vi "tiffWriteTags.vi"(6 "BitsPerSample":i32, 7 "Compress?":bool=TRUE, 8 "ImageDescription":string, 9 "Multipage":cluster{"Page":i32, "TotalPages":i32}, 10 "Dimensions":T1, 11 "TiffIn":refnum<k24>) -> (3 "TiffOut":refnum<k24>)   [LabVIEW 2012, in "LVTiffWriter.lvlib"]
uses:
  LVTiffWriter.lvlib
  D:/MyDocuments/LabVIEW Data/SPIM/Shared/libtiff.net_bin-2.4.500.0/BitMiracle.LibTiff.NET.dll
  BitMiracle.LibTiff.NET.dll
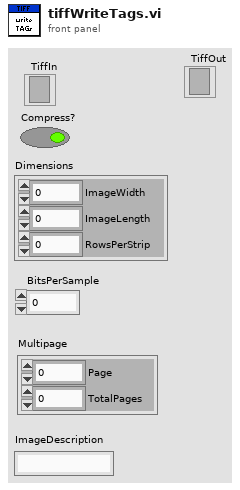
[diagram p1: front panel]
types:
  T1 = cluster{"ImageWidth":i32, "ImageLength":i32, "RowsPerStrip":i32}
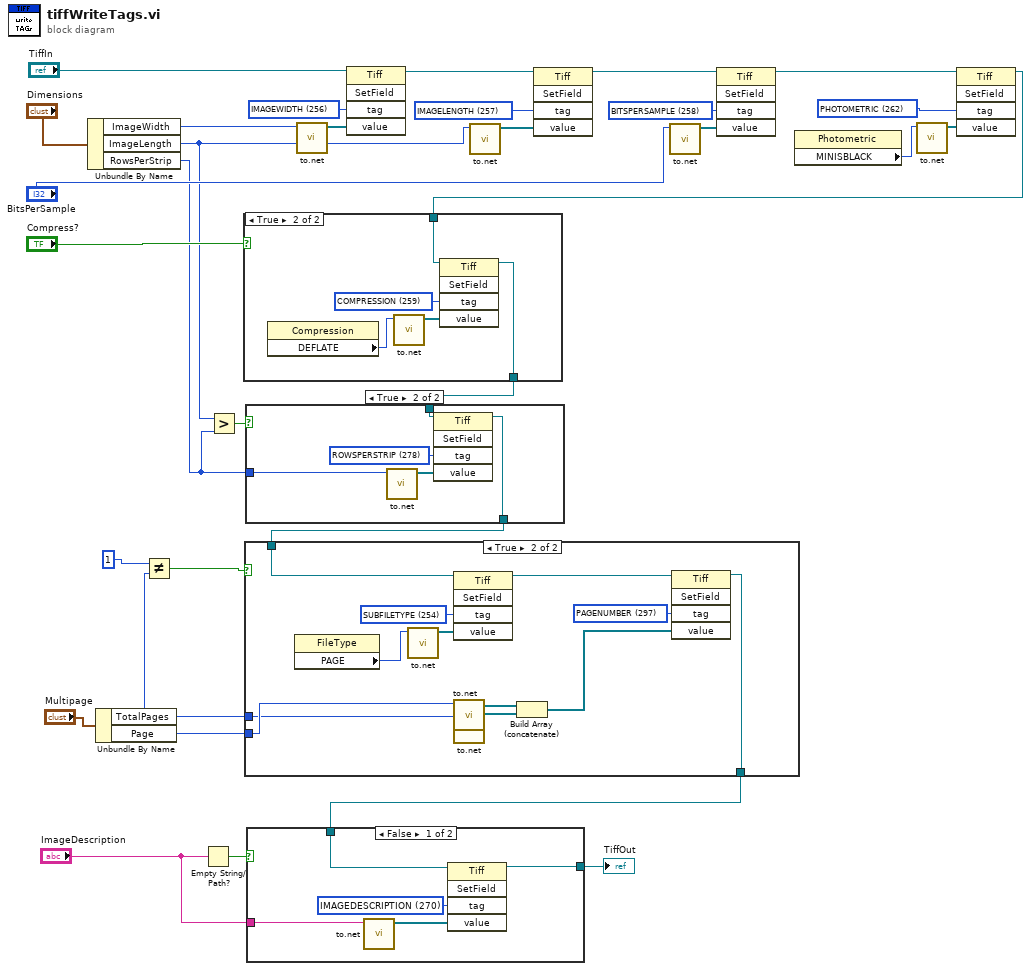
[diagram p0: block diagram]
diagram:
  w28 = 262 items=["IGNORE"=0, "SUBFILETYPE"=254, "OSUBFILETYPE"=255, "IMAGEWIDTH"=256, "IMAGELENGTH"=257, "BITSPERSAMPLE"=258, "COMPRESSION"=259, "PHOTOMETRIC"=262, "THRESHHOLDING"=263, "CELLWIDTH"=264, "CELLLENGTH"=265, "FILLORDER"=266, "DOCUMENTNAME"=269, "IMAGEDESCRIPTION"=270, "MAKE"=271, "MODEL"=272, "STRIPOFFSETS"=273, "ORIENTATION"=274, "SAMPLESPERPIXEL"=277, "ROWSPERSTRIP"=278, "STRIPBYTECOUNTS"=279, "MINSAMPLEVALUE"=280, "MAXSAMPLEVALUE"=281, "XRESOLUTION"=282, "YRESOLUTION"=283, "PLANARCONFIG"=284, "PAGENAME"=285, "XPOSITION"=286, "YPOSITION"=287, "FREEOFFSETS"=288, "FREEBYTECOUNTS"=289, "GRAYRESPONSEUNIT"=290, "GRAYRESPONSECURVE"=291, "GROUP3OPTIONS, T4OPTIONS"=292, "GROUP4OPTIONS, T6OPTIONS"=293, "RESOLUTIONUNIT"=296, "PAGENUMBER"=297, "COLORRESPONSEUNIT"=300, "TRANSFERFUNCTION"=301, "SOFTWARE"=305, "DATETIME"=306, "ARTIST"=315, "HOSTCOMPUTER"=316, "PREDICTOR"=317, "WHITEPOINT"=318, "PRIMARYCHROMATICITIES"=319, "COLORMAP"=320, "HALFTONEHINTS"=321, "TILEWIDTH"=322, "TILELENGTH"=323, "TILEOFFSETS"=324, "TILEBYTECOUNTS"=325, "BADFAXLINES"=326, "CLEANFAXDATA"=327, "CONSECUTIVEBADFAXLINES"=328, "SUBIFD"=330, "INKSET"=332, "INKNAMES"=333, "NUMBEROFINKS"=334, "DOTRANGE"=336, "TARGETPRINTER"=337, "EXTRASAMPLES"=338, "SAMPLEFORMAT"=339, "SMINSAMPLEVALUE"=340, "SMAXSAMPLEVALUE"=341, "CLIPPATH"=343, "XCLIPPATHUNITS"=344, "YCLIPPATHUNITS"=345, "INDEXED"=346, "JPEGTABLES"=347, "OPIPROXY"=351, "JPEGPROC"=512, "JPEGIFOFFSET"=513, "JPEGIFBYTECOUNT"=514, "JPEGRESTARTINTERVAL"=515, "JPEGLOSSLESSPREDICTORS"=517, "JPEGPOINTTRANSFORM"=518, "JPEGQTABLES"=519, "JPEGDCTABLES"=520, "JPEGACTABLES"=521, "YCBCRCOEFFICIENTS"=529, "YCBCRSUBSAMPLING"=530, "YCBCRPOSITIONING"=531, "REFERENCEBLACKWHITE"=532, "XMLPACKET"=700, "OPIIMAGEID"=32781, "REFPTS"=32953, "REGIONTACKPOINT"=32954, "REGIONWARPCORNERS"=32955, "REGIONAFFINE"=32956, "MATTEING"=32995, "DATATYPE"=32996, "IMAGEDEPTH"=32997, "TILEDEPTH"=32998, "PIXAR_IMAGEFULLWIDTH"=33300, "PIXAR_IMAGEFULLLENGTH"=33301, "PIXAR_TEXTUREFORMAT"=33302, "PIXAR_WRAPMODES"=33303, "PIXAR_FOVCOT"=33304, "PIXAR_MATRIX_WORLDTOSCREEN"=33305, "PIXAR_MATRIX_WORLDTOCAMERA"=33306, "WRITERSERIALNUMBER"=33405, "COPYRIGHT"=33432, "EXIF_EXPOSURETIME"=33434, "EXIF_FNUMBER"=33437, "RICHTIFFIPTC"=33723, "IT8SITE"=34016, "IT8COLORSEQUENCE"=34017, "IT8HEADER"=34018, "IT8RASTERPADDING"=34019, "IT8BITSPERRUNLENGTH"=34020, "IT8BITSPEREXTENDEDRUNLENGTH"=34021, "IT8COLORTABLE"=34022, "IT8IMAGECOLORINDICATOR"=34023, "IT8BKGCOLORINDICATOR"=34024, "IT8IMAGECOLORVALUE"=34025, "IT8BKGCOLORVALUE"=34026, "IT8PIXELINTENSITYRANGE"=34027, "IT8TRANSPARENCYINDICATOR"=34028, "IT8COLORCHARACTERIZATION"=34029, "IT8HCUSAGE"=34030, "IT8TRAPINDICATOR"=34031, "IT8CMYKEQUIVALENT"=34032, "FRAMECOUNT"=34232, "PHOTOSHOP"=34377, "EXIFIFD"=34665, "ICCPROFILE"=34675, "JBIGOPTIONS"=34750, "EXIF_EXPOSUREPROGRAM"=34850, "EXIF_SPECTRALSENSITIVITY"=34852, "GPSIFD"=34853, "EXIF_ISOSPEEDRATINGS"=34855, "EXIF_OECF"=34856, "FAXRECVPARAMS"=34908, "FAXSUBADDRESS"=34909, "FAXRECVTIME"=34910, "FAXDCS"=34911, "FEDEX_EDR"=34929, "EXIF_EXIFVERSION"=36864, "EXIF_DATETIMEORIGINAL"=36867, "EXIF_DATETIMEDIGITIZED"=36868, "EXIF_COMPONENTSCONFIGURATION"=37121, "EXIF_COMPRESSEDBITSPERPIXEL"=37122, "EXIF_SHUTTERSPEEDVALUE"=37377, "EXIF_APERTUREVALUE"=37378, "EXIF_BRIGHTNESSVALUE"=37379, "EXIF_EXPOSUREBIASVALUE"=37380, "EXIF_MAXAPERTUREVALUE"=37381, "EXIF_SUBJECTDISTANCE"=37382, "EXIF_METERINGMODE"=37383, "EXIF_LIGHTSOURCE"=37384, "EXIF_FLASH"=37385, "EXIF_FOCALLENGTH"=37386, "EXIF_SUBJECTAREA"=37396, "STONITS"=37439, "EXIF_MAKERNOTE"=37500, "EXIF_USERCOMMENT"=37510, "EXIF_SUBSECTIME"=37520, "EXIF_SUBSECTIMEORIGINAL"=37521, "EXIF_SUBSECTIMEDIGITIZED"=37522, "EXIF_FLASHPIXVERSION"=40960, "EXIF_COLORSPACE"=40961, "EXIF_PIXELXDIMENSION"=40962, "EXIF_PIXELYDIMENSION"=40963, "EXIF_RELATEDSOUNDFILE"=40964, "INTEROPERABILITYIFD"=40965, "EXIF_FLASHENERGY"=41483, "EXIF_SPATIALFREQUENCYRESPONSE"=41484, "EXIF_FOCALPLANEXRESOLUTION"=41486, "EXIF_FOCALPLANEYRESOLUTION"=41487, "EXIF_FOCALPLANERESOLUTIONUNIT"=41488, "EXIF_SUBJECTLOCATION"=41492, "EXIF_EXPOSUREINDEX"=41493, "EXIF_SENSINGMETHOD"=41495, "EXIF_FILESOURCE"=41728, "EXIF_SCENETYPE"=41729, "EXIF_CFAPATTERN"=41730, "EXIF_CUSTOMRENDERED"=41985, "EXIF_EXPOSUREMODE"=41986, "EXIF_WHITEBALANCE"=41987, "EXIF_DIGITALZOOMRATIO"=41988, "EXIF_FOCALLENGTHIN35MMFILM"=41989, "EXIF_SCENECAPTURETYPE"=41990, "EXIF_GAINCONTROL"=41991, "EXIF_CONTRAST"=41992, "EXIF_SATURATION"=41993, "EXIF_SHARPNESS"=41994, "EXIF_DEVICESETTINGDESCRIPTION"=41995, "EXIF_SUBJECTDISTANCERANGE"=41996, "EXIF_IMAGEUNIQUEID"=42016, "DNGVERSION"=50706, "DNGBACKWARDVERSION"=50707, "UNIQUECAMERAMODEL"=50708, "LOCALIZEDCAMERAMODEL"=50709, "CFAPLANECOLOR"=50710, "CFALAYOUT"=50711, "LINEARIZATIONTABLE"=50712, "BLACKLEVELREPEATDIM"=50713, "BLACKLEVEL"=50714, "BLACKLEVELDELTAH"=50715, "BLACKLEVELDELTAV"=50716, "WHITELEVEL"=50717, "DEFAULTSCALE"=50718, "DEFAULTCROPORIGIN"=50719, "DEFAULTCROPSIZE"=50720, "COLORMATRIX1"=50721, "COLORMATRIX2"=50722, "CAMERACALIBRATION1"=50723, "CAMERACALIBRATION2"=50724, "REDUCTIONMATRIX1"=50725, "REDUCTIONMATRIX2"=50726, "ANALOGBALANCE"=50727, "ASSHOTNEUTRAL"=50728, "ASSHOTWHITEXY"=50729, "BASELINEEXPOSURE"=50730, "BASELINENOISE"=50731, "BASELINESHARPNESS"=50732, "BAYERGREENSPLIT"=50733, "LINEARRESPONSELIMIT"=50734, "CAMERASERIALNUMBER"=50735, "LENSINFO"=50736, "CHROMABLURRADIUS"=50737, "ANTIALIASSTRENGTH"=50738, "SHADOWSCALE"=50739, "DNGPRIVATEDATA"=50740, "MAKERNOTESAFETY"=50741, "CALIBRATIONILLUMINANT1"=50778, "CALIBRATIONILLUMINANT2"=50779, "BESTQUALITYSCALE"=50780, "RAWDATAUNIQUEID"=50781, "ORIGINALRAWFILENAME"=50827, "ORIGINALRAWFILEDATA"=50828, "ACTIVEAREA"=50829, "MASKEDAREAS"=50830, "ASSHOTICCPROFILE"=50831, "ASSHOTPREPROFILEMATRIX"=50832, "CURRENTICCPROFILE"=50833, "CURRENTPREPROFILEMATRIX"=50834, "DCSHUESHIFTVALUES"=65535, "FAXMODE"=65536, "JPEGQUALITY"=65537, "JPEGCOLORMODE"=65538, "JPEGTABLESMODE"=65539, "FAXFILLFUNC"=65540, "PIXARLOGDATAFMT"=65549, "DCSIMAGERTYPE"=65550, "DCSINTERPMODE"=65551, "DCSBALANCEARRAY"=65552, "DCSCORRECTMATRIX"=65553, "DCSGAMMA"=65554, "DCSTOESHOULDERPTS"=65555, "DCSCALIBRATIONFD"=65556, "ZIPQUALITY"=65557, "PIXARLOGQUALITY"=65558, "DCSCLIPRECTANGLE"=65559, "SGILOGDATAFMT"=65560, "SGILOGENCODE"=65561] ("tag")
  w26 = 258 items=["IGNORE"=0, "SUBFILETYPE"=254, "OSUBFILETYPE"=255, "IMAGEWIDTH"=256, "IMAGELENGTH"=257, "BITSPERSAMPLE"=258, "COMPRESSION"=259, "PHOTOMETRIC"=262, "THRESHHOLDING"=263, "CELLWIDTH"=264, "CELLLENGTH"=265, "FILLORDER"=266, "DOCUMENTNAME"=269, "IMAGEDESCRIPTION"=270, "MAKE"=271, "MODEL"=272, "STRIPOFFSETS"=273, "ORIENTATION"=274, "SAMPLESPERPIXEL"=277, "ROWSPERSTRIP"=278, "STRIPBYTECOUNTS"=279, "MINSAMPLEVALUE"=280, "MAXSAMPLEVALUE"=281, "XRESOLUTION"=282, "YRESOLUTION"=283, "PLANARCONFIG"=284, "PAGENAME"=285, "XPOSITION"=286, "YPOSITION"=287, "FREEOFFSETS"=288, "FREEBYTECOUNTS"=289, "GRAYRESPONSEUNIT"=290, "GRAYRESPONSECURVE"=291, "GROUP3OPTIONS, T4OPTIONS"=292, "GROUP4OPTIONS, T6OPTIONS"=293, "RESOLUTIONUNIT"=296, "PAGENUMBER"=297, "COLORRESPONSEUNIT"=300, "TRANSFERFUNCTION"=301, "SOFTWARE"=305, "DATETIME"=306, "ARTIST"=315, "HOSTCOMPUTER"=316, "PREDICTOR"=317, "WHITEPOINT"=318, "PRIMARYCHROMATICITIES"=319, "COLORMAP"=320, "HALFTONEHINTS"=321, "TILEWIDTH"=322, "TILELENGTH"=323, "TILEOFFSETS"=324, "TILEBYTECOUNTS"=325, "BADFAXLINES"=326, "CLEANFAXDATA"=327, "CONSECUTIVEBADFAXLINES"=328, "SUBIFD"=330, "INKSET"=332, "INKNAMES"=333, "NUMBEROFINKS"=334, "DOTRANGE"=336, "TARGETPRINTER"=337, "EXTRASAMPLES"=338, "SAMPLEFORMAT"=339, "SMINSAMPLEVALUE"=340, "SMAXSAMPLEVALUE"=341, "CLIPPATH"=343, "XCLIPPATHUNITS"=344, "YCLIPPATHUNITS"=345, "INDEXED"=346, "JPEGTABLES"=347, "OPIPROXY"=351, "JPEGPROC"=512, "JPEGIFOFFSET"=513, "JPEGIFBYTECOUNT"=514, "JPEGRESTARTINTERVAL"=515, "JPEGLOSSLESSPREDICTORS"=517, "JPEGPOINTTRANSFORM"=518, "JPEGQTABLES"=519, "JPEGDCTABLES"=520, "JPEGACTABLES"=521, "YCBCRCOEFFICIENTS"=529, "YCBCRSUBSAMPLING"=530, "YCBCRPOSITIONING"=531, "REFERENCEBLACKWHITE"=532, "XMLPACKET"=700, "OPIIMAGEID"=32781, "REFPTS"=32953, "REGIONTACKPOINT"=32954, "REGIONWARPCORNERS"=32955, "REGIONAFFINE"=32956, "MATTEING"=32995, "DATATYPE"=32996, "IMAGEDEPTH"=32997, "TILEDEPTH"=32998, "PIXAR_IMAGEFULLWIDTH"=33300, "PIXAR_IMAGEFULLLENGTH"=33301, "PIXAR_TEXTUREFORMAT"=33302, "PIXAR_WRAPMODES"=33303, "PIXAR_FOVCOT"=33304, "PIXAR_MATRIX_WORLDTOSCREEN"=33305, "PIXAR_MATRIX_WORLDTOCAMERA"=33306, "WRITERSERIALNUMBER"=33405, "COPYRIGHT"=33432, "EXIF_EXPOSURETIME"=33434, "EXIF_FNUMBER"=33437, "RICHTIFFIPTC"=33723, "IT8SITE"=34016, "IT8COLORSEQUENCE"=34017, "IT8HEADER"=34018, "IT8RASTERPADDING"=34019, "IT8BITSPERRUNLENGTH"=34020, "IT8BITSPEREXTENDEDRUNLENGTH"=34021, "IT8COLORTABLE"=34022, "IT8IMAGECOLORINDICATOR"=34023, "IT8BKGCOLORINDICATOR"=34024, "IT8IMAGECOLORVALUE"=34025, "IT8BKGCOLORVALUE"=34026, "IT8PIXELINTENSITYRANGE"=34027, "IT8TRANSPARENCYINDICATOR"=34028, "IT8COLORCHARACTERIZATION"=34029, "IT8HCUSAGE"=34030, "IT8TRAPINDICATOR"=34031, "IT8CMYKEQUIVALENT"=34032, "FRAMECOUNT"=34232, "PHOTOSHOP"=34377, "EXIFIFD"=34665, "ICCPROFILE"=34675, "JBIGOPTIONS"=34750, "EXIF_EXPOSUREPROGRAM"=34850, "EXIF_SPECTRALSENSITIVITY"=34852, "GPSIFD"=34853, "EXIF_ISOSPEEDRATINGS"=34855, "EXIF_OECF"=34856, "FAXRECVPARAMS"=34908, "FAXSUBADDRESS"=34909, "FAXRECVTIME"=34910, "FAXDCS"=34911, "FEDEX_EDR"=34929, "EXIF_EXIFVERSION"=36864, "EXIF_DATETIMEORIGINAL"=36867, "EXIF_DATETIMEDIGITIZED"=36868, "EXIF_COMPONENTSCONFIGURATION"=37121, "EXIF_COMPRESSEDBITSPERPIXEL"=37122, "EXIF_SHUTTERSPEEDVALUE"=37377, "EXIF_APERTUREVALUE"=37378, "EXIF_BRIGHTNESSVALUE"=37379, "EXIF_EXPOSUREBIASVALUE"=37380, "EXIF_MAXAPERTUREVALUE"=37381, "EXIF_SUBJECTDISTANCE"=37382, "EXIF_METERINGMODE"=37383, "EXIF_LIGHTSOURCE"=37384, "EXIF_FLASH"=37385, "EXIF_FOCALLENGTH"=37386, "EXIF_SUBJECTAREA"=37396, "STONITS"=37439, "EXIF_MAKERNOTE"=37500, "EXIF_USERCOMMENT"=37510, "EXIF_SUBSECTIME"=37520, "EXIF_SUBSECTIMEORIGINAL"=37521, "EXIF_SUBSECTIMEDIGITIZED"=37522, "EXIF_FLASHPIXVERSION"=40960, "EXIF_COLORSPACE"=40961, "EXIF_PIXELXDIMENSION"=40962, "EXIF_PIXELYDIMENSION"=40963, "EXIF_RELATEDSOUNDFILE"=40964, "INTEROPERABILITYIFD"=40965, "EXIF_FLASHENERGY"=41483, "EXIF_SPATIALFREQUENCYRESPONSE"=41484, "EXIF_FOCALPLANEXRESOLUTION"=41486, "EXIF_FOCALPLANEYRESOLUTION"=41487, "EXIF_FOCALPLANERESOLUTIONUNIT"=41488, "EXIF_SUBJECTLOCATION"=41492, "EXIF_EXPOSUREINDEX"=41493, "EXIF_SENSINGMETHOD"=41495, "EXIF_FILESOURCE"=41728, "EXIF_SCENETYPE"=41729, "EXIF_CFAPATTERN"=41730, "EXIF_CUSTOMRENDERED"=41985, "EXIF_EXPOSUREMODE"=41986, "EXIF_WHITEBALANCE"=41987, "EXIF_DIGITALZOOMRATIO"=41988, "EXIF_FOCALLENGTHIN35MMFILM"=41989, "EXIF_SCENECAPTURETYPE"=41990, "EXIF_GAINCONTROL"=41991, "EXIF_CONTRAST"=41992, "EXIF_SATURATION"=41993, "EXIF_SHARPNESS"=41994, "EXIF_DEVICESETTINGDESCRIPTION"=41995, "EXIF_SUBJECTDISTANCERANGE"=41996, "EXIF_IMAGEUNIQUEID"=42016, "DNGVERSION"=50706, "DNGBACKWARDVERSION"=50707, "UNIQUECAMERAMODEL"=50708, "LOCALIZEDCAMERAMODEL"=50709, "CFAPLANECOLOR"=50710, "CFALAYOUT"=50711, "LINEARIZATIONTABLE"=50712, "BLACKLEVELREPEATDIM"=50713, "BLACKLEVEL"=50714, "BLACKLEVELDELTAH"=50715, "BLACKLEVELDELTAV"=50716, "WHITELEVEL"=50717, "DEFAULTSCALE"=50718, "DEFAULTCROPORIGIN"=50719, "DEFAULTCROPSIZE"=50720, "COLORMATRIX1"=50721, "COLORMATRIX2"=50722, "CAMERACALIBRATION1"=50723, "CAMERACALIBRATION2"=50724, "REDUCTIONMATRIX1"=50725, "REDUCTIONMATRIX2"=50726, "ANALOGBALANCE"=50727, "ASSHOTNEUTRAL"=50728, "ASSHOTWHITEXY"=50729, "BASELINEEXPOSURE"=50730, "BASELINENOISE"=50731, "BASELINESHARPNESS"=50732, "BAYERGREENSPLIT"=50733, "LINEARRESPONSELIMIT"=50734, "CAMERASERIALNUMBER"=50735, "LENSINFO"=50736, "CHROMABLURRADIUS"=50737, "ANTIALIASSTRENGTH"=50738, "SHADOWSCALE"=50739, "DNGPRIVATEDATA"=50740, "MAKERNOTESAFETY"=50741, "CALIBRATIONILLUMINANT1"=50778, "CALIBRATIONILLUMINANT2"=50779, "BESTQUALITYSCALE"=50780, "RAWDATAUNIQUEID"=50781, "ORIGINALRAWFILENAME"=50827, "ORIGINALRAWFILEDATA"=50828, "ACTIVEAREA"=50829, "MASKEDAREAS"=50830, "ASSHOTICCPROFILE"=50831, "ASSHOTPREPROFILEMATRIX"=50832, "CURRENTICCPROFILE"=50833, "CURRENTPREPROFILEMATRIX"=50834, "DCSHUESHIFTVALUES"=65535, "FAXMODE"=65536, "JPEGQUALITY"=65537, "JPEGCOLORMODE"=65538, "JPEGTABLESMODE"=65539, "FAXFILLFUNC"=65540, "PIXARLOGDATAFMT"=65549, "DCSIMAGERTYPE"=65550, "DCSINTERPMODE"=65551, "DCSBALANCEARRAY"=65552, "DCSCORRECTMATRIX"=65553, "DCSGAMMA"=65554, "DCSTOESHOULDERPTS"=65555, "DCSCALIBRATIONFD"=65556, "ZIPQUALITY"=65557, "PIXARLOGQUALITY"=65558, "DCSCLIPRECTANGLE"=65559, "SGILOGDATAFMT"=65560, "SGILOGENCODE"=65561] ("tag")
  w23 = 257 items=["IGNORE"=0, "SUBFILETYPE"=254, "OSUBFILETYPE"=255, "IMAGEWIDTH"=256, "IMAGELENGTH"=257, "BITSPERSAMPLE"=258, "COMPRESSION"=259, "PHOTOMETRIC"=262, "THRESHHOLDING"=263, "CELLWIDTH"=264, "CELLLENGTH"=265, "FILLORDER"=266, "DOCUMENTNAME"=269, "IMAGEDESCRIPTION"=270, "MAKE"=271, "MODEL"=272, "STRIPOFFSETS"=273, "ORIENTATION"=274, "SAMPLESPERPIXEL"=277, "ROWSPERSTRIP"=278, "STRIPBYTECOUNTS"=279, "MINSAMPLEVALUE"=280, "MAXSAMPLEVALUE"=281, "XRESOLUTION"=282, "YRESOLUTION"=283, "PLANARCONFIG"=284, "PAGENAME"=285, "XPOSITION"=286, "YPOSITION"=287, "FREEOFFSETS"=288, "FREEBYTECOUNTS"=289, "GRAYRESPONSEUNIT"=290, "GRAYRESPONSECURVE"=291, "GROUP3OPTIONS, T4OPTIONS"=292, "GROUP4OPTIONS, T6OPTIONS"=293, "RESOLUTIONUNIT"=296, "PAGENUMBER"=297, "COLORRESPONSEUNIT"=300, "TRANSFERFUNCTION"=301, "SOFTWARE"=305, "DATETIME"=306, "ARTIST"=315, "HOSTCOMPUTER"=316, "PREDICTOR"=317, "WHITEPOINT"=318, "PRIMARYCHROMATICITIES"=319, "COLORMAP"=320, "HALFTONEHINTS"=321, "TILEWIDTH"=322, "TILELENGTH"=323, "TILEOFFSETS"=324, "TILEBYTECOUNTS"=325, "BADFAXLINES"=326, "CLEANFAXDATA"=327, "CONSECUTIVEBADFAXLINES"=328, "SUBIFD"=330, "INKSET"=332, "INKNAMES"=333, "NUMBEROFINKS"=334, "DOTRANGE"=336, "TARGETPRINTER"=337, "EXTRASAMPLES"=338, "SAMPLEFORMAT"=339, "SMINSAMPLEVALUE"=340, "SMAXSAMPLEVALUE"=341, "CLIPPATH"=343, "XCLIPPATHUNITS"=344, "YCLIPPATHUNITS"=345, "INDEXED"=346, "JPEGTABLES"=347, "OPIPROXY"=351, "JPEGPROC"=512, "JPEGIFOFFSET"=513, "JPEGIFBYTECOUNT"=514, "JPEGRESTARTINTERVAL"=515, "JPEGLOSSLESSPREDICTORS"=517, "JPEGPOINTTRANSFORM"=518, "JPEGQTABLES"=519, "JPEGDCTABLES"=520, "JPEGACTABLES"=521, "YCBCRCOEFFICIENTS"=529, "YCBCRSUBSAMPLING"=530, "YCBCRPOSITIONING"=531, "REFERENCEBLACKWHITE"=532, "XMLPACKET"=700, "OPIIMAGEID"=32781, "REFPTS"=32953, "REGIONTACKPOINT"=32954, "REGIONWARPCORNERS"=32955, "REGIONAFFINE"=32956, "MATTEING"=32995, "DATATYPE"=32996, "IMAGEDEPTH"=32997, "TILEDEPTH"=32998, "PIXAR_IMAGEFULLWIDTH"=33300, "PIXAR_IMAGEFULLLENGTH"=33301, "PIXAR_TEXTUREFORMAT"=33302, "PIXAR_WRAPMODES"=33303, "PIXAR_FOVCOT"=33304, "PIXAR_MATRIX_WORLDTOSCREEN"=33305, "PIXAR_MATRIX_WORLDTOCAMERA"=33306, "WRITERSERIALNUMBER"=33405, "COPYRIGHT"=33432, "EXIF_EXPOSURETIME"=33434, "EXIF_FNUMBER"=33437, "RICHTIFFIPTC"=33723, "IT8SITE"=34016, "IT8COLORSEQUENCE"=34017, "IT8HEADER"=34018, "IT8RASTERPADDING"=34019, "IT8BITSPERRUNLENGTH"=34020, "IT8BITSPEREXTENDEDRUNLENGTH"=34021, "IT8COLORTABLE"=34022, "IT8IMAGECOLORINDICATOR"=34023, "IT8BKGCOLORINDICATOR"=34024, "IT8IMAGECOLORVALUE"=34025, "IT8BKGCOLORVALUE"=34026, "IT8PIXELINTENSITYRANGE"=34027, "IT8TRANSPARENCYINDICATOR"=34028, "IT8COLORCHARACTERIZATION"=34029, "IT8HCUSAGE"=34030, "IT8TRAPINDICATOR"=34031, "IT8CMYKEQUIVALENT"=34032, "FRAMECOUNT"=34232, "PHOTOSHOP"=34377, "EXIFIFD"=34665, "ICCPROFILE"=34675, "JBIGOPTIONS"=34750, "EXIF_EXPOSUREPROGRAM"=34850, "EXIF_SPECTRALSENSITIVITY"=34852, "GPSIFD"=34853, "EXIF_ISOSPEEDRATINGS"=34855, "EXIF_OECF"=34856, "FAXRECVPARAMS"=34908, "FAXSUBADDRESS"=34909, "FAXRECVTIME"=34910, "FAXDCS"=34911, "FEDEX_EDR"=34929, "EXIF_EXIFVERSION"=36864, "EXIF_DATETIMEORIGINAL"=36867, "EXIF_DATETIMEDIGITIZED"=36868, "EXIF_COMPONENTSCONFIGURATION"=37121, "EXIF_COMPRESSEDBITSPERPIXEL"=37122, "EXIF_SHUTTERSPEEDVALUE"=37377, "EXIF_APERTUREVALUE"=37378, "EXIF_BRIGHTNESSVALUE"=37379, "EXIF_EXPOSUREBIASVALUE"=37380, "EXIF_MAXAPERTUREVALUE"=37381, "EXIF_SUBJECTDISTANCE"=37382, "EXIF_METERINGMODE"=37383, "EXIF_LIGHTSOURCE"=37384, "EXIF_FLASH"=37385, "EXIF_FOCALLENGTH"=37386, "EXIF_SUBJECTAREA"=37396, "STONITS"=37439, "EXIF_MAKERNOTE"=37500, "EXIF_USERCOMMENT"=37510, "EXIF_SUBSECTIME"=37520, "EXIF_SUBSECTIMEORIGINAL"=37521, "EXIF_SUBSECTIMEDIGITIZED"=37522, "EXIF_FLASHPIXVERSION"=40960, "EXIF_COLORSPACE"=40961, "EXIF_PIXELXDIMENSION"=40962, "EXIF_PIXELYDIMENSION"=40963, "EXIF_RELATEDSOUNDFILE"=40964, "INTEROPERABILITYIFD"=40965, "EXIF_FLASHENERGY"=41483, "EXIF_SPATIALFREQUENCYRESPONSE"=41484, "EXIF_FOCALPLANEXRESOLUTION"=41486, "EXIF_FOCALPLANEYRESOLUTION"=41487, "EXIF_FOCALPLANERESOLUTIONUNIT"=41488, "EXIF_SUBJECTLOCATION"=41492, "EXIF_EXPOSUREINDEX"=41493, "EXIF_SENSINGMETHOD"=41495, "EXIF_FILESOURCE"=41728, "EXIF_SCENETYPE"=41729, "EXIF_CFAPATTERN"=41730, "EXIF_CUSTOMRENDERED"=41985, "EXIF_EXPOSUREMODE"=41986, "EXIF_WHITEBALANCE"=41987, "EXIF_DIGITALZOOMRATIO"=41988, "EXIF_FOCALLENGTHIN35MMFILM"=41989, "EXIF_SCENECAPTURETYPE"=41990, "EXIF_GAINCONTROL"=41991, "EXIF_CONTRAST"=41992, "EXIF_SATURATION"=41993, "EXIF_SHARPNESS"=41994, "EXIF_DEVICESETTINGDESCRIPTION"=41995, "EXIF_SUBJECTDISTANCERANGE"=41996, "EXIF_IMAGEUNIQUEID"=42016, "DNGVERSION"=50706, "DNGBACKWARDVERSION"=50707, "UNIQUECAMERAMODEL"=50708, "LOCALIZEDCAMERAMODEL"=50709, "CFAPLANECOLOR"=50710, "CFALAYOUT"=50711, "LINEARIZATIONTABLE"=50712, "BLACKLEVELREPEATDIM"=50713, "BLACKLEVEL"=50714, "BLACKLEVELDELTAH"=50715, "BLACKLEVELDELTAV"=50716, "WHITELEVEL"=50717, "DEFAULTSCALE"=50718, "DEFAULTCROPORIGIN"=50719, "DEFAULTCROPSIZE"=50720, "COLORMATRIX1"=50721, "COLORMATRIX2"=50722, "CAMERACALIBRATION1"=50723, "CAMERACALIBRATION2"=50724, "REDUCTIONMATRIX1"=50725, "REDUCTIONMATRIX2"=50726, "ANALOGBALANCE"=50727, "ASSHOTNEUTRAL"=50728, "ASSHOTWHITEXY"=50729, "BASELINEEXPOSURE"=50730, "BASELINENOISE"=50731, "BASELINESHARPNESS"=50732, "BAYERGREENSPLIT"=50733, "LINEARRESPONSELIMIT"=50734, "CAMERASERIALNUMBER"=50735, "LENSINFO"=50736, "CHROMABLURRADIUS"=50737, "ANTIALIASSTRENGTH"=50738, "SHADOWSCALE"=50739, "DNGPRIVATEDATA"=50740, "MAKERNOTESAFETY"=50741, "CALIBRATIONILLUMINANT1"=50778, "CALIBRATIONILLUMINANT2"=50779, "BESTQUALITYSCALE"=50780, "RAWDATAUNIQUEID"=50781, "ORIGINALRAWFILENAME"=50827, "ORIGINALRAWFILEDATA"=50828, "ACTIVEAREA"=50829, "MASKEDAREAS"=50830, "ASSHOTICCPROFILE"=50831, "ASSHOTPREPROFILEMATRIX"=50832, "CURRENTICCPROFILE"=50833, "CURRENTPREPROFILEMATRIX"=50834, "DCSHUESHIFTVALUES"=65535, "FAXMODE"=65536, "JPEGQUALITY"=65537, "JPEGCOLORMODE"=65538, "JPEGTABLESMODE"=65539, "FAXFILLFUNC"=65540, "PIXARLOGDATAFMT"=65549, "DCSIMAGERTYPE"=65550, "DCSINTERPMODE"=65551, "DCSBALANCEARRAY"=65552, "DCSCORRECTMATRIX"=65553, "DCSGAMMA"=65554, "DCSTOESHOULDERPTS"=65555, "DCSCALIBRATIONFD"=65556, "ZIPQUALITY"=65557, "PIXARLOGQUALITY"=65558, "DCSCLIPRECTANGLE"=65559, "SGILOGDATAFMT"=65560, "SGILOGENCODE"=65561] ("tag")
  w21 = 256 items=["IGNORE"=0, "SUBFILETYPE"=254, "OSUBFILETYPE"=255, "IMAGEWIDTH"=256, "IMAGELENGTH"=257, "BITSPERSAMPLE"=258, "COMPRESSION"=259, "PHOTOMETRIC"=262, "THRESHHOLDING"=263, "CELLWIDTH"=264, "CELLLENGTH"=265, "FILLORDER"=266, "DOCUMENTNAME"=269, "IMAGEDESCRIPTION"=270, "MAKE"=271, "MODEL"=272, "STRIPOFFSETS"=273, "ORIENTATION"=274, "SAMPLESPERPIXEL"=277, "ROWSPERSTRIP"=278, "STRIPBYTECOUNTS"=279, "MINSAMPLEVALUE"=280, "MAXSAMPLEVALUE"=281, "XRESOLUTION"=282, "YRESOLUTION"=283, "PLANARCONFIG"=284, "PAGENAME"=285, "XPOSITION"=286, "YPOSITION"=287, "FREEOFFSETS"=288, "FREEBYTECOUNTS"=289, "GRAYRESPONSEUNIT"=290, "GRAYRESPONSECURVE"=291, "GROUP3OPTIONS, T4OPTIONS"=292, "GROUP4OPTIONS, T6OPTIONS"=293, "RESOLUTIONUNIT"=296, "PAGENUMBER"=297, "COLORRESPONSEUNIT"=300, "TRANSFERFUNCTION"=301, "SOFTWARE"=305, "DATETIME"=306, "ARTIST"=315, "HOSTCOMPUTER"=316, "PREDICTOR"=317, "WHITEPOINT"=318, "PRIMARYCHROMATICITIES"=319, "COLORMAP"=320, "HALFTONEHINTS"=321, "TILEWIDTH"=322, "TILELENGTH"=323, "TILEOFFSETS"=324, "TILEBYTECOUNTS"=325, "BADFAXLINES"=326, "CLEANFAXDATA"=327, "CONSECUTIVEBADFAXLINES"=328, "SUBIFD"=330, "INKSET"=332, "INKNAMES"=333, "NUMBEROFINKS"=334, "DOTRANGE"=336, "TARGETPRINTER"=337, "EXTRASAMPLES"=338, "SAMPLEFORMAT"=339, "SMINSAMPLEVALUE"=340, "SMAXSAMPLEVALUE"=341, "CLIPPATH"=343, "XCLIPPATHUNITS"=344, "YCLIPPATHUNITS"=345, "INDEXED"=346, "JPEGTABLES"=347, "OPIPROXY"=351, "JPEGPROC"=512, "JPEGIFOFFSET"=513, "JPEGIFBYTECOUNT"=514, "JPEGRESTARTINTERVAL"=515, "JPEGLOSSLESSPREDICTORS"=517, "JPEGPOINTTRANSFORM"=518, "JPEGQTABLES"=519, "JPEGDCTABLES"=520, "JPEGACTABLES"=521, "YCBCRCOEFFICIENTS"=529, "YCBCRSUBSAMPLING"=530, "YCBCRPOSITIONING"=531, "REFERENCEBLACKWHITE"=532, "XMLPACKET"=700, "OPIIMAGEID"=32781, "REFPTS"=32953, "REGIONTACKPOINT"=32954, "REGIONWARPCORNERS"=32955, "REGIONAFFINE"=32956, "MATTEING"=32995, "DATATYPE"=32996, "IMAGEDEPTH"=32997, "TILEDEPTH"=32998, "PIXAR_IMAGEFULLWIDTH"=33300, "PIXAR_IMAGEFULLLENGTH"=33301, "PIXAR_TEXTUREFORMAT"=33302, "PIXAR_WRAPMODES"=33303, "PIXAR_FOVCOT"=33304, "PIXAR_MATRIX_WORLDTOSCREEN"=33305, "PIXAR_MATRIX_WORLDTOCAMERA"=33306, "WRITERSERIALNUMBER"=33405, "COPYRIGHT"=33432, "EXIF_EXPOSURETIME"=33434, "EXIF_FNUMBER"=33437, "RICHTIFFIPTC"=33723, "IT8SITE"=34016, "IT8COLORSEQUENCE"=34017, "IT8HEADER"=34018, "IT8RASTERPADDING"=34019, "IT8BITSPERRUNLENGTH"=34020, "IT8BITSPEREXTENDEDRUNLENGTH"=34021, "IT8COLORTABLE"=34022, "IT8IMAGECOLORINDICATOR"=34023, "IT8BKGCOLORINDICATOR"=34024, "IT8IMAGECOLORVALUE"=34025, "IT8BKGCOLORVALUE"=34026, "IT8PIXELINTENSITYRANGE"=34027, "IT8TRANSPARENCYINDICATOR"=34028, "IT8COLORCHARACTERIZATION"=34029, "IT8HCUSAGE"=34030, "IT8TRAPINDICATOR"=34031, "IT8CMYKEQUIVALENT"=34032, "FRAMECOUNT"=34232, "PHOTOSHOP"=34377, "EXIFIFD"=34665, "ICCPROFILE"=34675, "JBIGOPTIONS"=34750, "EXIF_EXPOSUREPROGRAM"=34850, "EXIF_SPECTRALSENSITIVITY"=34852, "GPSIFD"=34853, "EXIF_ISOSPEEDRATINGS"=34855, "EXIF_OECF"=34856, "FAXRECVPARAMS"=34908, "FAXSUBADDRESS"=34909, "FAXRECVTIME"=34910, "FAXDCS"=34911, "FEDEX_EDR"=34929, "EXIF_EXIFVERSION"=36864, "EXIF_DATETIMEORIGINAL"=36867, "EXIF_DATETIMEDIGITIZED"=36868, "EXIF_COMPONENTSCONFIGURATION"=37121, "EXIF_COMPRESSEDBITSPERPIXEL"=37122, "EXIF_SHUTTERSPEEDVALUE"=37377, "EXIF_APERTUREVALUE"=37378, "EXIF_BRIGHTNESSVALUE"=37379, "EXIF_EXPOSUREBIASVALUE"=37380, "EXIF_MAXAPERTUREVALUE"=37381, "EXIF_SUBJECTDISTANCE"=37382, "EXIF_METERINGMODE"=37383, "EXIF_LIGHTSOURCE"=37384, "EXIF_FLASH"=37385, "EXIF_FOCALLENGTH"=37386, "EXIF_SUBJECTAREA"=37396, "STONITS"=37439, "EXIF_MAKERNOTE"=37500, "EXIF_USERCOMMENT"=37510, "EXIF_SUBSECTIME"=37520, "EXIF_SUBSECTIMEORIGINAL"=37521, "EXIF_SUBSECTIMEDIGITIZED"=37522, "EXIF_FLASHPIXVERSION"=40960, "EXIF_COLORSPACE"=40961, "EXIF_PIXELXDIMENSION"=40962, "EXIF_PIXELYDIMENSION"=40963, "EXIF_RELATEDSOUNDFILE"=40964, "INTEROPERABILITYIFD"=40965, "EXIF_FLASHENERGY"=41483, "EXIF_SPATIALFREQUENCYRESPONSE"=41484, "EXIF_FOCALPLANEXRESOLUTION"=41486, "EXIF_FOCALPLANEYRESOLUTION"=41487, "EXIF_FOCALPLANERESOLUTIONUNIT"=41488, "EXIF_SUBJECTLOCATION"=41492, "EXIF_EXPOSUREINDEX"=41493, "EXIF_SENSINGMETHOD"=41495, "EXIF_FILESOURCE"=41728, "EXIF_SCENETYPE"=41729, "EXIF_CFAPATTERN"=41730, "EXIF_CUSTOMRENDERED"=41985, "EXIF_EXPOSUREMODE"=41986, "EXIF_WHITEBALANCE"=41987, "EXIF_DIGITALZOOMRATIO"=41988, "EXIF_FOCALLENGTHIN35MMFILM"=41989, "EXIF_SCENECAPTURETYPE"=41990, "EXIF_GAINCONTROL"=41991, "EXIF_CONTRAST"=41992, "EXIF_SATURATION"=41993, "EXIF_SHARPNESS"=41994, "EXIF_DEVICESETTINGDESCRIPTION"=41995, "EXIF_SUBJECTDISTANCERANGE"=41996, "EXIF_IMAGEUNIQUEID"=42016, "DNGVERSION"=50706, "DNGBACKWARDVERSION"=50707, "UNIQUECAMERAMODEL"=50708, "LOCALIZEDCAMERAMODEL"=50709, "CFAPLANECOLOR"=50710, "CFALAYOUT"=50711, "LINEARIZATIONTABLE"=50712, "BLACKLEVELREPEATDIM"=50713, "BLACKLEVEL"=50714, "BLACKLEVELDELTAH"=50715, "BLACKLEVELDELTAV"=50716, "WHITELEVEL"=50717, "DEFAULTSCALE"=50718, "DEFAULTCROPORIGIN"=50719, "DEFAULTCROPSIZE"=50720, "COLORMATRIX1"=50721, "COLORMATRIX2"=50722, "CAMERACALIBRATION1"=50723, "CAMERACALIBRATION2"=50724, "REDUCTIONMATRIX1"=50725, "REDUCTIONMATRIX2"=50726, "ANALOGBALANCE"=50727, "ASSHOTNEUTRAL"=50728, "ASSHOTWHITEXY"=50729, "BASELINEEXPOSURE"=50730, "BASELINENOISE"=50731, "BASELINESHARPNESS"=50732, "BAYERGREENSPLIT"=50733, "LINEARRESPONSELIMIT"=50734, "CAMERASERIALNUMBER"=50735, "LENSINFO"=50736, "CHROMABLURRADIUS"=50737, "ANTIALIASSTRENGTH"=50738, "SHADOWSCALE"=50739, "DNGPRIVATEDATA"=50740, "MAKERNOTESAFETY"=50741, "CALIBRATIONILLUMINANT1"=50778, "CALIBRATIONILLUMINANT2"=50779, "BESTQUALITYSCALE"=50780, "RAWDATAUNIQUEID"=50781, "ORIGINALRAWFILENAME"=50827, "ORIGINALRAWFILEDATA"=50828, "ACTIVEAREA"=50829, "MASKEDAREAS"=50830, "ASSHOTICCPROFILE"=50831, "ASSHOTPREPROFILEMATRIX"=50832, "CURRENTICCPROFILE"=50833, "CURRENTPREPROFILEMATRIX"=50834, "DCSHUESHIFTVALUES"=65535, "FAXMODE"=65536, "JPEGQUALITY"=65537, "JPEGCOLORMODE"=65538, "JPEGTABLESMODE"=65539, "FAXFILLFUNC"=65540, "PIXARLOGDATAFMT"=65549, "DCSIMAGERTYPE"=65550, "DCSINTERPMODE"=65551, "DCSBALANCEARRAY"=65552, "DCSCORRECTMATRIX"=65553, "DCSGAMMA"=65554, "DCSTOESHOULDERPTS"=65555, "DCSCALIBRATIONFD"=65556, "ZIPQUALITY"=65557, "PIXARLOGQUALITY"=65558, "DCSCLIPRECTANGLE"=65559, "SGILOGDATAFMT"=65560, "SGILOGENCODE"=65561] ("tag")
  n1 = Unbundle By Name("Dimensions") -> ("ImageWidth"=w13:i32, "ImageLength"=w12:i32, "RowsPerStrip"=w11:i32)
  n2 = Unbundle By Name("Multipage") -> ("TotalPages"=w7:i32, "Page"=w6:i32)
  n3 = Not Equal?(x=1 ("TotalPages"), y=w7) -> (x != y?=w10:bool)
  n4 = Empty String/Path?(string/path="ImageDescription") -> (empty?=w4:bool)
  n5 = Greater?(x=w12, y=w11) -> (0:w16:bool)
  n6 = call "to.net.vi"("Variant"=w13) -> ("Array"=w22:refnum<k24>[])  [unwired: 10 in]
  n7 = invoke class="Tiff" method="SetField"(reference="TiffIn", "tag"=w21, "value"=w22) -> (reference out=w25:refnum<k24>)  [unwired: 2 in, 4 out]
  n8 = call "to.net.vi"("Variant"=w12) -> ("Array"=w24:refnum<k24>[])  [unwired: 10 in]
  n9 = invoke class="Tiff" method="SetField"(reference=w25, "tag"=w23, "value"=w24) -> (reference out=w18:refnum<k24>)  [unwired: 2 in, 4 out]
  n10 = call "to.net.vi"("Variant"="BitsPerSample") -> ("Array"=w27:refnum<k24>[])  [unwired: 10 in]
  n11 = invoke class="Tiff" method="SetField"(reference=w18, "tag"=w26, "value"=w27) -> (reference out=w19:refnum<k24>)  [unwired: 2 in, 4 out]
  n12 = property class="Photometric"() -> ("MINISBLACK"=w30:i32)  [unwired: 2 in, 2 out]
  n13 = call "to.net.vi"("Variant"=w30) -> ("Array"=w29:refnum<k24>[])  [unwired: 10 in]
  n14 = invoke class="Tiff" method="SetField"(reference=w19, "tag"=w28, "value"=w29) -> (reference out=w31:refnum<k24>)  [unwired: 2 in, 4 out]
  n15 = case shown="True" "Compress?" {
    tunnel: w31 -> [w33 w38]
    tunnel: [w33 w34] -> w20
    frame False {
    }
    frame True {
      w35 = 259 items=["IGNORE"=0, "SUBFILETYPE"=254, "OSUBFILETYPE"=255, "IMAGEWIDTH"=256, "IMAGELENGTH"=257, "BITSPERSAMPLE"=258, "COMPRESSION"=259, "PHOTOMETRIC"=262, "THRESHHOLDING"=263, "CELLWIDTH"=264, "CELLLENGTH"=265, "FILLORDER"=266, "DOCUMENTNAME"=269, "IMAGEDESCRIPTION"=270, "MAKE"=271, "MODEL"=272, "STRIPOFFSETS"=273, "ORIENTATION"=274, "SAMPLESPERPIXEL"=277, "ROWSPERSTRIP"=278, "STRIPBYTECOUNTS"=279, "MINSAMPLEVALUE"=280, "MAXSAMPLEVALUE"=281, "XRESOLUTION"=282, "YRESOLUTION"=283, "PLANARCONFIG"=284, "PAGENAME"=285, "XPOSITION"=286, "YPOSITION"=287, "FREEOFFSETS"=288, "FREEBYTECOUNTS"=289, "GRAYRESPONSEUNIT"=290, "GRAYRESPONSECURVE"=291, "GROUP3OPTIONS, T4OPTIONS"=292, "GROUP4OPTIONS, T6OPTIONS"=293, "RESOLUTIONUNIT"=296, "PAGENUMBER"=297, "COLORRESPONSEUNIT"=300, "TRANSFERFUNCTION"=301, "SOFTWARE"=305, "DATETIME"=306, "ARTIST"=315, "HOSTCOMPUTER"=316, "PREDICTOR"=317, "WHITEPOINT"=318, "PRIMARYCHROMATICITIES"=319, "COLORMAP"=320, "HALFTONEHINTS"=321, "TILEWIDTH"=322, "TILELENGTH"=323, "TILEOFFSETS"=324, "TILEBYTECOUNTS"=325, "BADFAXLINES"=326, "CLEANFAXDATA"=327, "CONSECUTIVEBADFAXLINES"=328, "SUBIFD"=330, "INKSET"=332, "INKNAMES"=333, "NUMBEROFINKS"=334, "DOTRANGE"=336, "TARGETPRINTER"=337, "EXTRASAMPLES"=338, "SAMPLEFORMAT"=339, "SMINSAMPLEVALUE"=340, "SMAXSAMPLEVALUE"=341, "CLIPPATH"=343, "XCLIPPATHUNITS"=344, "YCLIPPATHUNITS"=345, "INDEXED"=346, "JPEGTABLES"=347, "OPIPROXY"=351, "JPEGPROC"=512, "JPEGIFOFFSET"=513, "JPEGIFBYTECOUNT"=514, "JPEGRESTARTINTERVAL"=515, "JPEGLOSSLESSPREDICTORS"=517, "JPEGPOINTTRANSFORM"=518, "JPEGQTABLES"=519, "JPEGDCTABLES"=520, "JPEGACTABLES"=521, "YCBCRCOEFFICIENTS"=529, "YCBCRSUBSAMPLING"=530, "YCBCRPOSITIONING"=531, "REFERENCEBLACKWHITE"=532, "XMLPACKET"=700, "OPIIMAGEID"=32781, "REFPTS"=32953, "REGIONTACKPOINT"=32954, "REGIONWARPCORNERS"=32955, "REGIONAFFINE"=32956, "MATTEING"=32995, "DATATYPE"=32996, "IMAGEDEPTH"=32997, "TILEDEPTH"=32998, "PIXAR_IMAGEFULLWIDTH"=33300, "PIXAR_IMAGEFULLLENGTH"=33301, "PIXAR_TEXTUREFORMAT"=33302, "PIXAR_WRAPMODES"=33303, "PIXAR_FOVCOT"=33304, "PIXAR_MATRIX_WORLDTOSCREEN"=33305, "PIXAR_MATRIX_WORLDTOCAMERA"=33306, "WRITERSERIALNUMBER"=33405, "COPYRIGHT"=33432, "EXIF_EXPOSURETIME"=33434, "EXIF_FNUMBER"=33437, "RICHTIFFIPTC"=33723, "IT8SITE"=34016, "IT8COLORSEQUENCE"=34017, "IT8HEADER"=34018, "IT8RASTERPADDING"=34019, "IT8BITSPERRUNLENGTH"=34020, "IT8BITSPEREXTENDEDRUNLENGTH"=34021, "IT8COLORTABLE"=34022, "IT8IMAGECOLORINDICATOR"=34023, "IT8BKGCOLORINDICATOR"=34024, "IT8IMAGECOLORVALUE"=34025, "IT8BKGCOLORVALUE"=34026, "IT8PIXELINTENSITYRANGE"=34027, "IT8TRANSPARENCYINDICATOR"=34028, "IT8COLORCHARACTERIZATION"=34029, "IT8HCUSAGE"=34030, "IT8TRAPINDICATOR"=34031, "IT8CMYKEQUIVALENT"=34032, "FRAMECOUNT"=34232, "PHOTOSHOP"=34377, "EXIFIFD"=34665, "ICCPROFILE"=34675, "JBIGOPTIONS"=34750, "EXIF_EXPOSUREPROGRAM"=34850, "EXIF_SPECTRALSENSITIVITY"=34852, "GPSIFD"=34853, "EXIF_ISOSPEEDRATINGS"=34855, "EXIF_OECF"=34856, "FAXRECVPARAMS"=34908, "FAXSUBADDRESS"=34909, "FAXRECVTIME"=34910, "FAXDCS"=34911, "FEDEX_EDR"=34929, "EXIF_EXIFVERSION"=36864, "EXIF_DATETIMEORIGINAL"=36867, "EXIF_DATETIMEDIGITIZED"=36868, "EXIF_COMPONENTSCONFIGURATION"=37121, "EXIF_COMPRESSEDBITSPERPIXEL"=37122, "EXIF_SHUTTERSPEEDVALUE"=37377, "EXIF_APERTUREVALUE"=37378, "EXIF_BRIGHTNESSVALUE"=37379, "EXIF_EXPOSUREBIASVALUE"=37380, "EXIF_MAXAPERTUREVALUE"=37381, "EXIF_SUBJECTDISTANCE"=37382, "EXIF_METERINGMODE"=37383, "EXIF_LIGHTSOURCE"=37384, "EXIF_FLASH"=37385, "EXIF_FOCALLENGTH"=37386, "EXIF_SUBJECTAREA"=37396, "STONITS"=37439, "EXIF_MAKERNOTE"=37500, "EXIF_USERCOMMENT"=37510, "EXIF_SUBSECTIME"=37520, "EXIF_SUBSECTIMEORIGINAL"=37521, "EXIF_SUBSECTIMEDIGITIZED"=37522, "EXIF_FLASHPIXVERSION"=40960, "EXIF_COLORSPACE"=40961, "EXIF_PIXELXDIMENSION"=40962, "EXIF_PIXELYDIMENSION"=40963, "EXIF_RELATEDSOUNDFILE"=40964, "INTEROPERABILITYIFD"=40965, "EXIF_FLASHENERGY"=41483, "EXIF_SPATIALFREQUENCYRESPONSE"=41484, "EXIF_FOCALPLANEXRESOLUTION"=41486, "EXIF_FOCALPLANEYRESOLUTION"=41487, "EXIF_FOCALPLANERESOLUTIONUNIT"=41488, "EXIF_SUBJECTLOCATION"=41492, "EXIF_EXPOSUREINDEX"=41493, "EXIF_SENSINGMETHOD"=41495, "EXIF_FILESOURCE"=41728, "EXIF_SCENETYPE"=41729, "EXIF_CFAPATTERN"=41730, "EXIF_CUSTOMRENDERED"=41985, "EXIF_EXPOSUREMODE"=41986, "EXIF_WHITEBALANCE"=41987, "EXIF_DIGITALZOOMRATIO"=41988, "EXIF_FOCALLENGTHIN35MMFILM"=41989, "EXIF_SCENECAPTURETYPE"=41990, "EXIF_GAINCONTROL"=41991, "EXIF_CONTRAST"=41992, "EXIF_SATURATION"=41993, "EXIF_SHARPNESS"=41994, "EXIF_DEVICESETTINGDESCRIPTION"=41995, "EXIF_SUBJECTDISTANCERANGE"=41996, "EXIF_IMAGEUNIQUEID"=42016, "DNGVERSION"=50706, "DNGBACKWARDVERSION"=50707, "UNIQUECAMERAMODEL"=50708, "LOCALIZEDCAMERAMODEL"=50709, "CFAPLANECOLOR"=50710, "CFALAYOUT"=50711, "LINEARIZATIONTABLE"=50712, "BLACKLEVELREPEATDIM"=50713, "BLACKLEVEL"=50714, "BLACKLEVELDELTAH"=50715, "BLACKLEVELDELTAV"=50716, "WHITELEVEL"=50717, "DEFAULTSCALE"=50718, "DEFAULTCROPORIGIN"=50719, "DEFAULTCROPSIZE"=50720, "COLORMATRIX1"=50721, "COLORMATRIX2"=50722, "CAMERACALIBRATION1"=50723, "CAMERACALIBRATION2"=50724, "REDUCTIONMATRIX1"=50725, "REDUCTIONMATRIX2"=50726, "ANALOGBALANCE"=50727, "ASSHOTNEUTRAL"=50728, "ASSHOTWHITEXY"=50729, "BASELINEEXPOSURE"=50730, "BASELINENOISE"=50731, "BASELINESHARPNESS"=50732, "BAYERGREENSPLIT"=50733, "LINEARRESPONSELIMIT"=50734, "CAMERASERIALNUMBER"=50735, "LENSINFO"=50736, "CHROMABLURRADIUS"=50737, "ANTIALIASSTRENGTH"=50738, "SHADOWSCALE"=50739, "DNGPRIVATEDATA"=50740, "MAKERNOTESAFETY"=50741, "CALIBRATIONILLUMINANT1"=50778, "CALIBRATIONILLUMINANT2"=50779, "BESTQUALITYSCALE"=50780, "RAWDATAUNIQUEID"=50781, "ORIGINALRAWFILENAME"=50827, "ORIGINALRAWFILEDATA"=50828, "ACTIVEAREA"=50829, "MASKEDAREAS"=50830, "ASSHOTICCPROFILE"=50831, "ASSHOTPREPROFILEMATRIX"=50832, "CURRENTICCPROFILE"=50833, "CURRENTPREPROFILEMATRIX"=50834, "DCSHUESHIFTVALUES"=65535, "FAXMODE"=65536, "JPEGQUALITY"=65537, "JPEGCOLORMODE"=65538, "JPEGTABLESMODE"=65539, "FAXFILLFUNC"=65540, "PIXARLOGDATAFMT"=65549, "DCSIMAGERTYPE"=65550, "DCSINTERPMODE"=65551, "DCSBALANCEARRAY"=65552, "DCSCORRECTMATRIX"=65553, "DCSGAMMA"=65554, "DCSTOESHOULDERPTS"=65555, "DCSCALIBRATIONFD"=65556, "ZIPQUALITY"=65557, "PIXARLOGQUALITY"=65558, "DCSCLIPRECTANGLE"=65559, "SGILOGDATAFMT"=65560, "SGILOGENCODE"=65561] ("tag")
      n16 = property class="Compression"() -> ("DEFLATE"=w37:i32)  [unwired: 2 in, 2 out]
      n17 = call "to.net.vi"("Variant"=w37) -> ("Array"=w36:refnum<k24>[])  [unwired: 10 in]
      n18 = invoke class="Tiff" method="SetField"(reference=w38, "tag"=w35, "value"=w36) -> (reference out=w34:refnum<k24>)  [unwired: 2 in, 4 out]
    }
  }
  n19 = case shown="True" w16 {
    tunnel: [w39 w42] -> w5
    tunnel: w20 -> [w39 w41]
    tunnel: w11 -> [_ w40]
    frame False {
    }
    frame True {
      w43 = 278 items=["IGNORE"=0, "SUBFILETYPE"=254, "OSUBFILETYPE"=255, "IMAGEWIDTH"=256, "IMAGELENGTH"=257, "BITSPERSAMPLE"=258, "COMPRESSION"=259, "PHOTOMETRIC"=262, "THRESHHOLDING"=263, "CELLWIDTH"=264, "CELLLENGTH"=265, "FILLORDER"=266, "DOCUMENTNAME"=269, "IMAGEDESCRIPTION"=270, "MAKE"=271, "MODEL"=272, "STRIPOFFSETS"=273, "ORIENTATION"=274, "SAMPLESPERPIXEL"=277, "ROWSPERSTRIP"=278, "STRIPBYTECOUNTS"=279, "MINSAMPLEVALUE"=280, "MAXSAMPLEVALUE"=281, "XRESOLUTION"=282, "YRESOLUTION"=283, "PLANARCONFIG"=284, "PAGENAME"=285, "XPOSITION"=286, "YPOSITION"=287, "FREEOFFSETS"=288, "FREEBYTECOUNTS"=289, "GRAYRESPONSEUNIT"=290, "GRAYRESPONSECURVE"=291, "GROUP3OPTIONS, T4OPTIONS"=292, "GROUP4OPTIONS, T6OPTIONS"=293, "RESOLUTIONUNIT"=296, "PAGENUMBER"=297, "COLORRESPONSEUNIT"=300, "TRANSFERFUNCTION"=301, "SOFTWARE"=305, "DATETIME"=306, "ARTIST"=315, "HOSTCOMPUTER"=316, "PREDICTOR"=317, "WHITEPOINT"=318, "PRIMARYCHROMATICITIES"=319, "COLORMAP"=320, "HALFTONEHINTS"=321, "TILEWIDTH"=322, "TILELENGTH"=323, "TILEOFFSETS"=324, "TILEBYTECOUNTS"=325, "BADFAXLINES"=326, "CLEANFAXDATA"=327, "CONSECUTIVEBADFAXLINES"=328, "SUBIFD"=330, "INKSET"=332, "INKNAMES"=333, "NUMBEROFINKS"=334, "DOTRANGE"=336, "TARGETPRINTER"=337, "EXTRASAMPLES"=338, "SAMPLEFORMAT"=339, "SMINSAMPLEVALUE"=340, "SMAXSAMPLEVALUE"=341, "CLIPPATH"=343, "XCLIPPATHUNITS"=344, "YCLIPPATHUNITS"=345, "INDEXED"=346, "JPEGTABLES"=347, "OPIPROXY"=351, "JPEGPROC"=512, "JPEGIFOFFSET"=513, "JPEGIFBYTECOUNT"=514, "JPEGRESTARTINTERVAL"=515, "JPEGLOSSLESSPREDICTORS"=517, "JPEGPOINTTRANSFORM"=518, "JPEGQTABLES"=519, "JPEGDCTABLES"=520, "JPEGACTABLES"=521, "YCBCRCOEFFICIENTS"=529, "YCBCRSUBSAMPLING"=530, "YCBCRPOSITIONING"=531, "REFERENCEBLACKWHITE"=532, "XMLPACKET"=700, "OPIIMAGEID"=32781, "REFPTS"=32953, "REGIONTACKPOINT"=32954, "REGIONWARPCORNERS"=32955, "REGIONAFFINE"=32956, "MATTEING"=32995, "DATATYPE"=32996, "IMAGEDEPTH"=32997, "TILEDEPTH"=32998, "PIXAR_IMAGEFULLWIDTH"=33300, "PIXAR_IMAGEFULLLENGTH"=33301, "PIXAR_TEXTUREFORMAT"=33302, "PIXAR_WRAPMODES"=33303, "PIXAR_FOVCOT"=33304, "PIXAR_MATRIX_WORLDTOSCREEN"=33305, "PIXAR_MATRIX_WORLDTOCAMERA"=33306, "WRITERSERIALNUMBER"=33405, "COPYRIGHT"=33432, "EXIF_EXPOSURETIME"=33434, "EXIF_FNUMBER"=33437, "RICHTIFFIPTC"=33723, "IT8SITE"=34016, "IT8COLORSEQUENCE"=34017, "IT8HEADER"=34018, "IT8RASTERPADDING"=34019, "IT8BITSPERRUNLENGTH"=34020, "IT8BITSPEREXTENDEDRUNLENGTH"=34021, "IT8COLORTABLE"=34022, "IT8IMAGECOLORINDICATOR"=34023, "IT8BKGCOLORINDICATOR"=34024, "IT8IMAGECOLORVALUE"=34025, "IT8BKGCOLORVALUE"=34026, "IT8PIXELINTENSITYRANGE"=34027, "IT8TRANSPARENCYINDICATOR"=34028, "IT8COLORCHARACTERIZATION"=34029, "IT8HCUSAGE"=34030, "IT8TRAPINDICATOR"=34031, "IT8CMYKEQUIVALENT"=34032, "FRAMECOUNT"=34232, "PHOTOSHOP"=34377, "EXIFIFD"=34665, "ICCPROFILE"=34675, "JBIGOPTIONS"=34750, "EXIF_EXPOSUREPROGRAM"=34850, "EXIF_SPECTRALSENSITIVITY"=34852, "GPSIFD"=34853, "EXIF_ISOSPEEDRATINGS"=34855, "EXIF_OECF"=34856, "FAXRECVPARAMS"=34908, "FAXSUBADDRESS"=34909, "FAXRECVTIME"=34910, "FAXDCS"=34911, "FEDEX_EDR"=34929, "EXIF_EXIFVERSION"=36864, "EXIF_DATETIMEORIGINAL"=36867, "EXIF_DATETIMEDIGITIZED"=36868, "EXIF_COMPONENTSCONFIGURATION"=37121, "EXIF_COMPRESSEDBITSPERPIXEL"=37122, "EXIF_SHUTTERSPEEDVALUE"=37377, "EXIF_APERTUREVALUE"=37378, "EXIF_BRIGHTNESSVALUE"=37379, "EXIF_EXPOSUREBIASVALUE"=37380, "EXIF_MAXAPERTUREVALUE"=37381, "EXIF_SUBJECTDISTANCE"=37382, "EXIF_METERINGMODE"=37383, "EXIF_LIGHTSOURCE"=37384, "EXIF_FLASH"=37385, "EXIF_FOCALLENGTH"=37386, "EXIF_SUBJECTAREA"=37396, "STONITS"=37439, "EXIF_MAKERNOTE"=37500, "EXIF_USERCOMMENT"=37510, "EXIF_SUBSECTIME"=37520, "EXIF_SUBSECTIMEORIGINAL"=37521, "EXIF_SUBSECTIMEDIGITIZED"=37522, "EXIF_FLASHPIXVERSION"=40960, "EXIF_COLORSPACE"=40961, "EXIF_PIXELXDIMENSION"=40962, "EXIF_PIXELYDIMENSION"=40963, "EXIF_RELATEDSOUNDFILE"=40964, "INTEROPERABILITYIFD"=40965, "EXIF_FLASHENERGY"=41483, "EXIF_SPATIALFREQUENCYRESPONSE"=41484, "EXIF_FOCALPLANEXRESOLUTION"=41486, "EXIF_FOCALPLANEYRESOLUTION"=41487, "EXIF_FOCALPLANERESOLUTIONUNIT"=41488, "EXIF_SUBJECTLOCATION"=41492, "EXIF_EXPOSUREINDEX"=41493, "EXIF_SENSINGMETHOD"=41495, "EXIF_FILESOURCE"=41728, "EXIF_SCENETYPE"=41729, "EXIF_CFAPATTERN"=41730, "EXIF_CUSTOMRENDERED"=41985, "EXIF_EXPOSUREMODE"=41986, "EXIF_WHITEBALANCE"=41987, "EXIF_DIGITALZOOMRATIO"=41988, "EXIF_FOCALLENGTHIN35MMFILM"=41989, "EXIF_SCENECAPTURETYPE"=41990, "EXIF_GAINCONTROL"=41991, "EXIF_CONTRAST"=41992, "EXIF_SATURATION"=41993, "EXIF_SHARPNESS"=41994, "EXIF_DEVICESETTINGDESCRIPTION"=41995, "EXIF_SUBJECTDISTANCERANGE"=41996, "EXIF_IMAGEUNIQUEID"=42016, "DNGVERSION"=50706, "DNGBACKWARDVERSION"=50707, "UNIQUECAMERAMODEL"=50708, "LOCALIZEDCAMERAMODEL"=50709, "CFAPLANECOLOR"=50710, "CFALAYOUT"=50711, "LINEARIZATIONTABLE"=50712, "BLACKLEVELREPEATDIM"=50713, "BLACKLEVEL"=50714, "BLACKLEVELDELTAH"=50715, "BLACKLEVELDELTAV"=50716, "WHITELEVEL"=50717, "DEFAULTSCALE"=50718, "DEFAULTCROPORIGIN"=50719, "DEFAULTCROPSIZE"=50720, "COLORMATRIX1"=50721, "COLORMATRIX2"=50722, "CAMERACALIBRATION1"=50723, "CAMERACALIBRATION2"=50724, "REDUCTIONMATRIX1"=50725, "REDUCTIONMATRIX2"=50726, "ANALOGBALANCE"=50727, "ASSHOTNEUTRAL"=50728, "ASSHOTWHITEXY"=50729, "BASELINEEXPOSURE"=50730, "BASELINENOISE"=50731, "BASELINESHARPNESS"=50732, "BAYERGREENSPLIT"=50733, "LINEARRESPONSELIMIT"=50734, "CAMERASERIALNUMBER"=50735, "LENSINFO"=50736, "CHROMABLURRADIUS"=50737, "ANTIALIASSTRENGTH"=50738, "SHADOWSCALE"=50739, "DNGPRIVATEDATA"=50740, "MAKERNOTESAFETY"=50741, "CALIBRATIONILLUMINANT1"=50778, "CALIBRATIONILLUMINANT2"=50779, "BESTQUALITYSCALE"=50780, "RAWDATAUNIQUEID"=50781, "ORIGINALRAWFILENAME"=50827, "ORIGINALRAWFILEDATA"=50828, "ACTIVEAREA"=50829, "MASKEDAREAS"=50830, "ASSHOTICCPROFILE"=50831, "ASSHOTPREPROFILEMATRIX"=50832, "CURRENTICCPROFILE"=50833, "CURRENTPREPROFILEMATRIX"=50834, "DCSHUESHIFTVALUES"=65535, "FAXMODE"=65536, "JPEGQUALITY"=65537, "JPEGCOLORMODE"=65538, "JPEGTABLESMODE"=65539, "FAXFILLFUNC"=65540, "PIXARLOGDATAFMT"=65549, "DCSIMAGERTYPE"=65550, "DCSINTERPMODE"=65551, "DCSBALANCEARRAY"=65552, "DCSCORRECTMATRIX"=65553, "DCSGAMMA"=65554, "DCSTOESHOULDERPTS"=65555, "DCSCALIBRATIONFD"=65556, "ZIPQUALITY"=65557, "PIXARLOGQUALITY"=65558, "DCSCLIPRECTANGLE"=65559, "SGILOGDATAFMT"=65560, "SGILOGENCODE"=65561] ("tag")
      n20 = call "to.net.vi"("Variant"=w40) -> ("Array"=w44:refnum<k24>[])  [unwired: 10 in]
      n21 = invoke class="Tiff" method="SetField"(reference=w41, "tag"=w43, "value"=w44) -> (reference out=w42:refnum<k24>)  [unwired: 2 in, 4 out]
    }
  }
  n22 = case shown="True" w10 {
    tunnel: w7 -> [_ w51]
    tunnel: w6 -> [_ w52]
    tunnel: w5 -> [w45 w46]
    tunnel: [w45 w56] -> w2
    frame False {
    }
    frame True {
      w53 = 254 items=["IGNORE"=0, "SUBFILETYPE"=254, "OSUBFILETYPE"=255, "IMAGEWIDTH"=256, "IMAGELENGTH"=257, "BITSPERSAMPLE"=258, "COMPRESSION"=259, "PHOTOMETRIC"=262, "THRESHHOLDING"=263, "CELLWIDTH"=264, "CELLLENGTH"=265, "FILLORDER"=266, "DOCUMENTNAME"=269, "IMAGEDESCRIPTION"=270, "MAKE"=271, "MODEL"=272, "STRIPOFFSETS"=273, "ORIENTATION"=274, "SAMPLESPERPIXEL"=277, "ROWSPERSTRIP"=278, "STRIPBYTECOUNTS"=279, "MINSAMPLEVALUE"=280, "MAXSAMPLEVALUE"=281, "XRESOLUTION"=282, "YRESOLUTION"=283, "PLANARCONFIG"=284, "PAGENAME"=285, "XPOSITION"=286, "YPOSITION"=287, "FREEOFFSETS"=288, "FREEBYTECOUNTS"=289, "GRAYRESPONSEUNIT"=290, "GRAYRESPONSECURVE"=291, "GROUP3OPTIONS, T4OPTIONS"=292, "GROUP4OPTIONS, T6OPTIONS"=293, "RESOLUTIONUNIT"=296, "PAGENUMBER"=297, "COLORRESPONSEUNIT"=300, "TRANSFERFUNCTION"=301, "SOFTWARE"=305, "DATETIME"=306, "ARTIST"=315, "HOSTCOMPUTER"=316, "PREDICTOR"=317, "WHITEPOINT"=318, "PRIMARYCHROMATICITIES"=319, "COLORMAP"=320, "HALFTONEHINTS"=321, "TILEWIDTH"=322, "TILELENGTH"=323, "TILEOFFSETS"=324, "TILEBYTECOUNTS"=325, "BADFAXLINES"=326, "CLEANFAXDATA"=327, "CONSECUTIVEBADFAXLINES"=328, "SUBIFD"=330, "INKSET"=332, "INKNAMES"=333, "NUMBEROFINKS"=334, "DOTRANGE"=336, "TARGETPRINTER"=337, "EXTRASAMPLES"=338, "SAMPLEFORMAT"=339, "SMINSAMPLEVALUE"=340, "SMAXSAMPLEVALUE"=341, "CLIPPATH"=343, "XCLIPPATHUNITS"=344, "YCLIPPATHUNITS"=345, "INDEXED"=346, "JPEGTABLES"=347, "OPIPROXY"=351, "JPEGPROC"=512, "JPEGIFOFFSET"=513, "JPEGIFBYTECOUNT"=514, "JPEGRESTARTINTERVAL"=515, "JPEGLOSSLESSPREDICTORS"=517, "JPEGPOINTTRANSFORM"=518, "JPEGQTABLES"=519, "JPEGDCTABLES"=520, "JPEGACTABLES"=521, "YCBCRCOEFFICIENTS"=529, "YCBCRSUBSAMPLING"=530, "YCBCRPOSITIONING"=531, "REFERENCEBLACKWHITE"=532, "XMLPACKET"=700, "OPIIMAGEID"=32781, "REFPTS"=32953, "REGIONTACKPOINT"=32954, "REGIONWARPCORNERS"=32955, "REGIONAFFINE"=32956, "MATTEING"=32995, "DATATYPE"=32996, "IMAGEDEPTH"=32997, "TILEDEPTH"=32998, "PIXAR_IMAGEFULLWIDTH"=33300, "PIXAR_IMAGEFULLLENGTH"=33301, "PIXAR_TEXTUREFORMAT"=33302, "PIXAR_WRAPMODES"=33303, "PIXAR_FOVCOT"=33304, "PIXAR_MATRIX_WORLDTOSCREEN"=33305, "PIXAR_MATRIX_WORLDTOCAMERA"=33306, "WRITERSERIALNUMBER"=33405, "COPYRIGHT"=33432, "EXIF_EXPOSURETIME"=33434, "EXIF_FNUMBER"=33437, "RICHTIFFIPTC"=33723, "IT8SITE"=34016, "IT8COLORSEQUENCE"=34017, "IT8HEADER"=34018, "IT8RASTERPADDING"=34019, "IT8BITSPERRUNLENGTH"=34020, "IT8BITSPEREXTENDEDRUNLENGTH"=34021, "IT8COLORTABLE"=34022, "IT8IMAGECOLORINDICATOR"=34023, "IT8BKGCOLORINDICATOR"=34024, "IT8IMAGECOLORVALUE"=34025, "IT8BKGCOLORVALUE"=34026, "IT8PIXELINTENSITYRANGE"=34027, "IT8TRANSPARENCYINDICATOR"=34028, "IT8COLORCHARACTERIZATION"=34029, "IT8HCUSAGE"=34030, "IT8TRAPINDICATOR"=34031, "IT8CMYKEQUIVALENT"=34032, "FRAMECOUNT"=34232, "PHOTOSHOP"=34377, "EXIFIFD"=34665, "ICCPROFILE"=34675, "JBIGOPTIONS"=34750, "EXIF_EXPOSUREPROGRAM"=34850, "EXIF_SPECTRALSENSITIVITY"=34852, "GPSIFD"=34853, "EXIF_ISOSPEEDRATINGS"=34855, "EXIF_OECF"=34856, "FAXRECVPARAMS"=34908, "FAXSUBADDRESS"=34909, "FAXRECVTIME"=34910, "FAXDCS"=34911, "FEDEX_EDR"=34929, "EXIF_EXIFVERSION"=36864, "EXIF_DATETIMEORIGINAL"=36867, "EXIF_DATETIMEDIGITIZED"=36868, "EXIF_COMPONENTSCONFIGURATION"=37121, "EXIF_COMPRESSEDBITSPERPIXEL"=37122, "EXIF_SHUTTERSPEEDVALUE"=37377, "EXIF_APERTUREVALUE"=37378, "EXIF_BRIGHTNESSVALUE"=37379, "EXIF_EXPOSUREBIASVALUE"=37380, "EXIF_MAXAPERTUREVALUE"=37381, "EXIF_SUBJECTDISTANCE"=37382, "EXIF_METERINGMODE"=37383, "EXIF_LIGHTSOURCE"=37384, "EXIF_FLASH"=37385, "EXIF_FOCALLENGTH"=37386, "EXIF_SUBJECTAREA"=37396, "STONITS"=37439, "EXIF_MAKERNOTE"=37500, "EXIF_USERCOMMENT"=37510, "EXIF_SUBSECTIME"=37520, "EXIF_SUBSECTIMEORIGINAL"=37521, "EXIF_SUBSECTIMEDIGITIZED"=37522, "EXIF_FLASHPIXVERSION"=40960, "EXIF_COLORSPACE"=40961, "EXIF_PIXELXDIMENSION"=40962, "EXIF_PIXELYDIMENSION"=40963, "EXIF_RELATEDSOUNDFILE"=40964, "INTEROPERABILITYIFD"=40965, "EXIF_FLASHENERGY"=41483, "EXIF_SPATIALFREQUENCYRESPONSE"=41484, "EXIF_FOCALPLANEXRESOLUTION"=41486, "EXIF_FOCALPLANEYRESOLUTION"=41487, "EXIF_FOCALPLANERESOLUTIONUNIT"=41488, "EXIF_SUBJECTLOCATION"=41492, "EXIF_EXPOSUREINDEX"=41493, "EXIF_SENSINGMETHOD"=41495, "EXIF_FILESOURCE"=41728, "EXIF_SCENETYPE"=41729, "EXIF_CFAPATTERN"=41730, "EXIF_CUSTOMRENDERED"=41985, "EXIF_EXPOSUREMODE"=41986, "EXIF_WHITEBALANCE"=41987, "EXIF_DIGITALZOOMRATIO"=41988, "EXIF_FOCALLENGTHIN35MMFILM"=41989, "EXIF_SCENECAPTURETYPE"=41990, "EXIF_GAINCONTROL"=41991, "EXIF_CONTRAST"=41992, "EXIF_SATURATION"=41993, "EXIF_SHARPNESS"=41994, "EXIF_DEVICESETTINGDESCRIPTION"=41995, "EXIF_SUBJECTDISTANCERANGE"=41996, "EXIF_IMAGEUNIQUEID"=42016, "DNGVERSION"=50706, "DNGBACKWARDVERSION"=50707, "UNIQUECAMERAMODEL"=50708, "LOCALIZEDCAMERAMODEL"=50709, "CFAPLANECOLOR"=50710, "CFALAYOUT"=50711, "LINEARIZATIONTABLE"=50712, "BLACKLEVELREPEATDIM"=50713, "BLACKLEVEL"=50714, "BLACKLEVELDELTAH"=50715, "BLACKLEVELDELTAV"=50716, "WHITELEVEL"=50717, "DEFAULTSCALE"=50718, "DEFAULTCROPORIGIN"=50719, "DEFAULTCROPSIZE"=50720, "COLORMATRIX1"=50721, "COLORMATRIX2"=50722, "CAMERACALIBRATION1"=50723, "CAMERACALIBRATION2"=50724, "REDUCTIONMATRIX1"=50725, "REDUCTIONMATRIX2"=50726, "ANALOGBALANCE"=50727, "ASSHOTNEUTRAL"=50728, "ASSHOTWHITEXY"=50729, "BASELINEEXPOSURE"=50730, "BASELINENOISE"=50731, "BASELINESHARPNESS"=50732, "BAYERGREENSPLIT"=50733, "LINEARRESPONSELIMIT"=50734, "CAMERASERIALNUMBER"=50735, "LENSINFO"=50736, "CHROMABLURRADIUS"=50737, "ANTIALIASSTRENGTH"=50738, "SHADOWSCALE"=50739, "DNGPRIVATEDATA"=50740, "MAKERNOTESAFETY"=50741, "CALIBRATIONILLUMINANT1"=50778, "CALIBRATIONILLUMINANT2"=50779, "BESTQUALITYSCALE"=50780, "RAWDATAUNIQUEID"=50781, "ORIGINALRAWFILENAME"=50827, "ORIGINALRAWFILEDATA"=50828, "ACTIVEAREA"=50829, "MASKEDAREAS"=50830, "ASSHOTICCPROFILE"=50831, "ASSHOTPREPROFILEMATRIX"=50832, "CURRENTICCPROFILE"=50833, "CURRENTPREPROFILEMATRIX"=50834, "DCSHUESHIFTVALUES"=65535, "FAXMODE"=65536, "JPEGQUALITY"=65537, "JPEGCOLORMODE"=65538, "JPEGTABLESMODE"=65539, "FAXFILLFUNC"=65540, "PIXARLOGDATAFMT"=65549, "DCSIMAGERTYPE"=65550, "DCSINTERPMODE"=65551, "DCSBALANCEARRAY"=65552, "DCSCORRECTMATRIX"=65553, "DCSGAMMA"=65554, "DCSTOESHOULDERPTS"=65555, "DCSCALIBRATIONFD"=65556, "ZIPQUALITY"=65557, "PIXARLOGQUALITY"=65558, "DCSCLIPRECTANGLE"=65559, "SGILOGDATAFMT"=65560, "SGILOGENCODE"=65561] ("tag")
      w57 = 297 items=["IGNORE"=0, "SUBFILETYPE"=254, "OSUBFILETYPE"=255, "IMAGEWIDTH"=256, "IMAGELENGTH"=257, "BITSPERSAMPLE"=258, "COMPRESSION"=259, "PHOTOMETRIC"=262, "THRESHHOLDING"=263, "CELLWIDTH"=264, "CELLLENGTH"=265, "FILLORDER"=266, "DOCUMENTNAME"=269, "IMAGEDESCRIPTION"=270, "MAKE"=271, "MODEL"=272, "STRIPOFFSETS"=273, "ORIENTATION"=274, "SAMPLESPERPIXEL"=277, "ROWSPERSTRIP"=278, "STRIPBYTECOUNTS"=279, "MINSAMPLEVALUE"=280, "MAXSAMPLEVALUE"=281, "XRESOLUTION"=282, "YRESOLUTION"=283, "PLANARCONFIG"=284, "PAGENAME"=285, "XPOSITION"=286, "YPOSITION"=287, "FREEOFFSETS"=288, "FREEBYTECOUNTS"=289, "GRAYRESPONSEUNIT"=290, "GRAYRESPONSECURVE"=291, "GROUP3OPTIONS, T4OPTIONS"=292, "GROUP4OPTIONS, T6OPTIONS"=293, "RESOLUTIONUNIT"=296, "PAGENUMBER"=297, "COLORRESPONSEUNIT"=300, "TRANSFERFUNCTION"=301, "SOFTWARE"=305, "DATETIME"=306, "ARTIST"=315, "HOSTCOMPUTER"=316, "PREDICTOR"=317, "WHITEPOINT"=318, "PRIMARYCHROMATICITIES"=319, "COLORMAP"=320, "HALFTONEHINTS"=321, "TILEWIDTH"=322, "TILELENGTH"=323, "TILEOFFSETS"=324, "TILEBYTECOUNTS"=325, "BADFAXLINES"=326, "CLEANFAXDATA"=327, "CONSECUTIVEBADFAXLINES"=328, "SUBIFD"=330, "INKSET"=332, "INKNAMES"=333, "NUMBEROFINKS"=334, "DOTRANGE"=336, "TARGETPRINTER"=337, "EXTRASAMPLES"=338, "SAMPLEFORMAT"=339, "SMINSAMPLEVALUE"=340, "SMAXSAMPLEVALUE"=341, "CLIPPATH"=343, "XCLIPPATHUNITS"=344, "YCLIPPATHUNITS"=345, "INDEXED"=346, "JPEGTABLES"=347, "OPIPROXY"=351, "JPEGPROC"=512, "JPEGIFOFFSET"=513, "JPEGIFBYTECOUNT"=514, "JPEGRESTARTINTERVAL"=515, "JPEGLOSSLESSPREDICTORS"=517, "JPEGPOINTTRANSFORM"=518, "JPEGQTABLES"=519, "JPEGDCTABLES"=520, "JPEGACTABLES"=521, "YCBCRCOEFFICIENTS"=529, "YCBCRSUBSAMPLING"=530, "YCBCRPOSITIONING"=531, "REFERENCEBLACKWHITE"=532, "XMLPACKET"=700, "OPIIMAGEID"=32781, "REFPTS"=32953, "REGIONTACKPOINT"=32954, "REGIONWARPCORNERS"=32955, "REGIONAFFINE"=32956, "MATTEING"=32995, "DATATYPE"=32996, "IMAGEDEPTH"=32997, "TILEDEPTH"=32998, "PIXAR_IMAGEFULLWIDTH"=33300, "PIXAR_IMAGEFULLLENGTH"=33301, "PIXAR_TEXTUREFORMAT"=33302, "PIXAR_WRAPMODES"=33303, "PIXAR_FOVCOT"=33304, "PIXAR_MATRIX_WORLDTOSCREEN"=33305, "PIXAR_MATRIX_WORLDTOCAMERA"=33306, "WRITERSERIALNUMBER"=33405, "COPYRIGHT"=33432, "EXIF_EXPOSURETIME"=33434, "EXIF_FNUMBER"=33437, "RICHTIFFIPTC"=33723, "IT8SITE"=34016, "IT8COLORSEQUENCE"=34017, "IT8HEADER"=34018, "IT8RASTERPADDING"=34019, "IT8BITSPERRUNLENGTH"=34020, "IT8BITSPEREXTENDEDRUNLENGTH"=34021, "IT8COLORTABLE"=34022, "IT8IMAGECOLORINDICATOR"=34023, "IT8BKGCOLORINDICATOR"=34024, "IT8IMAGECOLORVALUE"=34025, "IT8BKGCOLORVALUE"=34026, "IT8PIXELINTENSITYRANGE"=34027, "IT8TRANSPARENCYINDICATOR"=34028, "IT8COLORCHARACTERIZATION"=34029, "IT8HCUSAGE"=34030, "IT8TRAPINDICATOR"=34031, "IT8CMYKEQUIVALENT"=34032, "FRAMECOUNT"=34232, "PHOTOSHOP"=34377, "EXIFIFD"=34665, "ICCPROFILE"=34675, "JBIGOPTIONS"=34750, "EXIF_EXPOSUREPROGRAM"=34850, "EXIF_SPECTRALSENSITIVITY"=34852, "GPSIFD"=34853, "EXIF_ISOSPEEDRATINGS"=34855, "EXIF_OECF"=34856, "FAXRECVPARAMS"=34908, "FAXSUBADDRESS"=34909, "FAXRECVTIME"=34910, "FAXDCS"=34911, "FEDEX_EDR"=34929, "EXIF_EXIFVERSION"=36864, "EXIF_DATETIMEORIGINAL"=36867, "EXIF_DATETIMEDIGITIZED"=36868, "EXIF_COMPONENTSCONFIGURATION"=37121, "EXIF_COMPRESSEDBITSPERPIXEL"=37122, "EXIF_SHUTTERSPEEDVALUE"=37377, "EXIF_APERTUREVALUE"=37378, "EXIF_BRIGHTNESSVALUE"=37379, "EXIF_EXPOSUREBIASVALUE"=37380, "EXIF_MAXAPERTUREVALUE"=37381, "EXIF_SUBJECTDISTANCE"=37382, "EXIF_METERINGMODE"=37383, "EXIF_LIGHTSOURCE"=37384, "EXIF_FLASH"=37385, "EXIF_FOCALLENGTH"=37386, "EXIF_SUBJECTAREA"=37396, "STONITS"=37439, "EXIF_MAKERNOTE"=37500, "EXIF_USERCOMMENT"=37510, "EXIF_SUBSECTIME"=37520, "EXIF_SUBSECTIMEORIGINAL"=37521, "EXIF_SUBSECTIMEDIGITIZED"=37522, "EXIF_FLASHPIXVERSION"=40960, "EXIF_COLORSPACE"=40961, "EXIF_PIXELXDIMENSION"=40962, "EXIF_PIXELYDIMENSION"=40963, "EXIF_RELATEDSOUNDFILE"=40964, "INTEROPERABILITYIFD"=40965, "EXIF_FLASHENERGY"=41483, "EXIF_SPATIALFREQUENCYRESPONSE"=41484, "EXIF_FOCALPLANEXRESOLUTION"=41486, "EXIF_FOCALPLANEYRESOLUTION"=41487, "EXIF_FOCALPLANERESOLUTIONUNIT"=41488, "EXIF_SUBJECTLOCATION"=41492, "EXIF_EXPOSUREINDEX"=41493, "EXIF_SENSINGMETHOD"=41495, "EXIF_FILESOURCE"=41728, "EXIF_SCENETYPE"=41729, "EXIF_CFAPATTERN"=41730, "EXIF_CUSTOMRENDERED"=41985, "EXIF_EXPOSUREMODE"=41986, "EXIF_WHITEBALANCE"=41987, "EXIF_DIGITALZOOMRATIO"=41988, "EXIF_FOCALLENGTHIN35MMFILM"=41989, "EXIF_SCENECAPTURETYPE"=41990, "EXIF_GAINCONTROL"=41991, "EXIF_CONTRAST"=41992, "EXIF_SATURATION"=41993, "EXIF_SHARPNESS"=41994, "EXIF_DEVICESETTINGDESCRIPTION"=41995, "EXIF_SUBJECTDISTANCERANGE"=41996, "EXIF_IMAGEUNIQUEID"=42016, "DNGVERSION"=50706, "DNGBACKWARDVERSION"=50707, "UNIQUECAMERAMODEL"=50708, "LOCALIZEDCAMERAMODEL"=50709, "CFAPLANECOLOR"=50710, "CFALAYOUT"=50711, "LINEARIZATIONTABLE"=50712, "BLACKLEVELREPEATDIM"=50713, "BLACKLEVEL"=50714, "BLACKLEVELDELTAH"=50715, "BLACKLEVELDELTAV"=50716, "WHITELEVEL"=50717, "DEFAULTSCALE"=50718, "DEFAULTCROPORIGIN"=50719, "DEFAULTCROPSIZE"=50720, "COLORMATRIX1"=50721, "COLORMATRIX2"=50722, "CAMERACALIBRATION1"=50723, "CAMERACALIBRATION2"=50724, "REDUCTIONMATRIX1"=50725, "REDUCTIONMATRIX2"=50726, "ANALOGBALANCE"=50727, "ASSHOTNEUTRAL"=50728, "ASSHOTWHITEXY"=50729, "BASELINEEXPOSURE"=50730, "BASELINENOISE"=50731, "BASELINESHARPNESS"=50732, "BAYERGREENSPLIT"=50733, "LINEARRESPONSELIMIT"=50734, "CAMERASERIALNUMBER"=50735, "LENSINFO"=50736, "CHROMABLURRADIUS"=50737, "ANTIALIASSTRENGTH"=50738, "SHADOWSCALE"=50739, "DNGPRIVATEDATA"=50740, "MAKERNOTESAFETY"=50741, "CALIBRATIONILLUMINANT1"=50778, "CALIBRATIONILLUMINANT2"=50779, "BESTQUALITYSCALE"=50780, "RAWDATAUNIQUEID"=50781, "ORIGINALRAWFILENAME"=50827, "ORIGINALRAWFILEDATA"=50828, "ACTIVEAREA"=50829, "MASKEDAREAS"=50830, "ASSHOTICCPROFILE"=50831, "ASSHOTPREPROFILEMATRIX"=50832, "CURRENTICCPROFILE"=50833, "CURRENTPREPROFILEMATRIX"=50834, "DCSHUESHIFTVALUES"=65535, "FAXMODE"=65536, "JPEGQUALITY"=65537, "JPEGCOLORMODE"=65538, "JPEGTABLESMODE"=65539, "FAXFILLFUNC"=65540, "PIXARLOGDATAFMT"=65549, "DCSIMAGERTYPE"=65550, "DCSINTERPMODE"=65551, "DCSBALANCEARRAY"=65552, "DCSCORRECTMATRIX"=65553, "DCSGAMMA"=65554, "DCSTOESHOULDERPTS"=65555, "DCSCALIBRATIONFD"=65556, "ZIPQUALITY"=65557, "PIXARLOGQUALITY"=65558, "DCSCLIPRECTANGLE"=65559, "SGILOGDATAFMT"=65560, "SGILOGENCODE"=65561] ("tag")
      n23 = property class="FileType"() -> ("PAGE"=w55:i32)  [unwired: 2 in, 2 out]
      n24 = call "to.net.vi"("Variant"=w55) -> ("Array"=w54:refnum<k24>[])  [unwired: 10 in]
      n25 = invoke class="Tiff" method="SetField"(reference=w46, "tag"=w53, "value"=w54) -> (reference out=w47:refnum<k24>)  [unwired: 2 in, 4 out]
      n26 = call "to.net.vi"("Variant"=w52) -> ("Array"=w50:refnum<k24>[])  [unwired: 10 in]
      n27 = call "to.net.vi"("Variant"=w51) -> ("Array"=w49:refnum<k24>[])  [unwired: 10 in]
      n28 = Build Array (concatenate)(w50, w49) -> (w48:refnum<k24>[])
      n29 = invoke class="Tiff" method="SetField"(reference=w47, "tag"=w57, "value"=w48) -> (reference out=w56:refnum<k24>)  [unwired: 2 in, 4 out]
    }
  }
  n30 = case shown="False" w4 {
    tunnel: "ImageDescription" -> [w59 _]
    tunnel: w2 -> [w61 w63]
    tunnel: [w58 w63] -> w1
    frame False {
      w62 = 270 items=["IGNORE"=0, "SUBFILETYPE"=254, "OSUBFILETYPE"=255, "IMAGEWIDTH"=256, "IMAGELENGTH"=257, "BITSPERSAMPLE"=258, "COMPRESSION"=259, "PHOTOMETRIC"=262, "THRESHHOLDING"=263, "CELLWIDTH"=264, "CELLLENGTH"=265, "FILLORDER"=266, "DOCUMENTNAME"=269, "IMAGEDESCRIPTION"=270, "MAKE"=271, "MODEL"=272, "STRIPOFFSETS"=273, "ORIENTATION"=274, "SAMPLESPERPIXEL"=277, "ROWSPERSTRIP"=278, "STRIPBYTECOUNTS"=279, "MINSAMPLEVALUE"=280, "MAXSAMPLEVALUE"=281, "XRESOLUTION"=282, "YRESOLUTION"=283, "PLANARCONFIG"=284, "PAGENAME"=285, "XPOSITION"=286, "YPOSITION"=287, "FREEOFFSETS"=288, "FREEBYTECOUNTS"=289, "GRAYRESPONSEUNIT"=290, "GRAYRESPONSECURVE"=291, "GROUP3OPTIONS, T4OPTIONS"=292, "GROUP4OPTIONS, T6OPTIONS"=293, "RESOLUTIONUNIT"=296, "PAGENUMBER"=297, "COLORRESPONSEUNIT"=300, "TRANSFERFUNCTION"=301, "SOFTWARE"=305, "DATETIME"=306, "ARTIST"=315, "HOSTCOMPUTER"=316, "PREDICTOR"=317, "WHITEPOINT"=318, "PRIMARYCHROMATICITIES"=319, "COLORMAP"=320, "HALFTONEHINTS"=321, "TILEWIDTH"=322, "TILELENGTH"=323, "TILEOFFSETS"=324, "TILEBYTECOUNTS"=325, "BADFAXLINES"=326, "CLEANFAXDATA"=327, "CONSECUTIVEBADFAXLINES"=328, "SUBIFD"=330, "INKSET"=332, "INKNAMES"=333, "NUMBEROFINKS"=334, "DOTRANGE"=336, "TARGETPRINTER"=337, "EXTRASAMPLES"=338, "SAMPLEFORMAT"=339, "SMINSAMPLEVALUE"=340, "SMAXSAMPLEVALUE"=341, "CLIPPATH"=343, "XCLIPPATHUNITS"=344, "YCLIPPATHUNITS"=345, "INDEXED"=346, "JPEGTABLES"=347, "OPIPROXY"=351, "JPEGPROC"=512, "JPEGIFOFFSET"=513, "JPEGIFBYTECOUNT"=514, "JPEGRESTARTINTERVAL"=515, "JPEGLOSSLESSPREDICTORS"=517, "JPEGPOINTTRANSFORM"=518, "JPEGQTABLES"=519, "JPEGDCTABLES"=520, "JPEGACTABLES"=521, "YCBCRCOEFFICIENTS"=529, "YCBCRSUBSAMPLING"=530, "YCBCRPOSITIONING"=531, "REFERENCEBLACKWHITE"=532, "XMLPACKET"=700, "OPIIMAGEID"=32781, "REFPTS"=32953, "REGIONTACKPOINT"=32954, "REGIONWARPCORNERS"=32955, "REGIONAFFINE"=32956, "MATTEING"=32995, "DATATYPE"=32996, "IMAGEDEPTH"=32997, "TILEDEPTH"=32998, "PIXAR_IMAGEFULLWIDTH"=33300, "PIXAR_IMAGEFULLLENGTH"=33301, "PIXAR_TEXTUREFORMAT"=33302, "PIXAR_WRAPMODES"=33303, "PIXAR_FOVCOT"=33304, "PIXAR_MATRIX_WORLDTOSCREEN"=33305, "PIXAR_MATRIX_WORLDTOCAMERA"=33306, "WRITERSERIALNUMBER"=33405, "COPYRIGHT"=33432, "EXIF_EXPOSURETIME"=33434, "EXIF_FNUMBER"=33437, "RICHTIFFIPTC"=33723, "IT8SITE"=34016, "IT8COLORSEQUENCE"=34017, "IT8HEADER"=34018, "IT8RASTERPADDING"=34019, "IT8BITSPERRUNLENGTH"=34020, "IT8BITSPEREXTENDEDRUNLENGTH"=34021, "IT8COLORTABLE"=34022, "IT8IMAGECOLORINDICATOR"=34023, "IT8BKGCOLORINDICATOR"=34024, "IT8IMAGECOLORVALUE"=34025, "IT8BKGCOLORVALUE"=34026, "IT8PIXELINTENSITYRANGE"=34027, "IT8TRANSPARENCYINDICATOR"=34028, "IT8COLORCHARACTERIZATION"=34029, "IT8HCUSAGE"=34030, "IT8TRAPINDICATOR"=34031, "IT8CMYKEQUIVALENT"=34032, "FRAMECOUNT"=34232, "PHOTOSHOP"=34377, "EXIFIFD"=34665, "ICCPROFILE"=34675, "JBIGOPTIONS"=34750, "EXIF_EXPOSUREPROGRAM"=34850, "EXIF_SPECTRALSENSITIVITY"=34852, "GPSIFD"=34853, "EXIF_ISOSPEEDRATINGS"=34855, "EXIF_OECF"=34856, "FAXRECVPARAMS"=34908, "FAXSUBADDRESS"=34909, "FAXRECVTIME"=34910, "FAXDCS"=34911, "FEDEX_EDR"=34929, "EXIF_EXIFVERSION"=36864, "EXIF_DATETIMEORIGINAL"=36867, "EXIF_DATETIMEDIGITIZED"=36868, "EXIF_COMPONENTSCONFIGURATION"=37121, "EXIF_COMPRESSEDBITSPERPIXEL"=37122, "EXIF_SHUTTERSPEEDVALUE"=37377, "EXIF_APERTUREVALUE"=37378, "EXIF_BRIGHTNESSVALUE"=37379, "EXIF_EXPOSUREBIASVALUE"=37380, "EXIF_MAXAPERTUREVALUE"=37381, "EXIF_SUBJECTDISTANCE"=37382, "EXIF_METERINGMODE"=37383, "EXIF_LIGHTSOURCE"=37384, "EXIF_FLASH"=37385, "EXIF_FOCALLENGTH"=37386, "EXIF_SUBJECTAREA"=37396, "STONITS"=37439, "EXIF_MAKERNOTE"=37500, "EXIF_USERCOMMENT"=37510, "EXIF_SUBSECTIME"=37520, "EXIF_SUBSECTIMEORIGINAL"=37521, "EXIF_SUBSECTIMEDIGITIZED"=37522, "EXIF_FLASHPIXVERSION"=40960, "EXIF_COLORSPACE"=40961, "EXIF_PIXELXDIMENSION"=40962, "EXIF_PIXELYDIMENSION"=40963, "EXIF_RELATEDSOUNDFILE"=40964, "INTEROPERABILITYIFD"=40965, "EXIF_FLASHENERGY"=41483, "EXIF_SPATIALFREQUENCYRESPONSE"=41484, "EXIF_FOCALPLANEXRESOLUTION"=41486, "EXIF_FOCALPLANEYRESOLUTION"=41487, "EXIF_FOCALPLANERESOLUTIONUNIT"=41488, "EXIF_SUBJECTLOCATION"=41492, "EXIF_EXPOSUREINDEX"=41493, "EXIF_SENSINGMETHOD"=41495, "EXIF_FILESOURCE"=41728, "EXIF_SCENETYPE"=41729, "EXIF_CFAPATTERN"=41730, "EXIF_CUSTOMRENDERED"=41985, "EXIF_EXPOSUREMODE"=41986, "EXIF_WHITEBALANCE"=41987, "EXIF_DIGITALZOOMRATIO"=41988, "EXIF_FOCALLENGTHIN35MMFILM"=41989, "EXIF_SCENECAPTURETYPE"=41990, "EXIF_GAINCONTROL"=41991, "EXIF_CONTRAST"=41992, "EXIF_SATURATION"=41993, "EXIF_SHARPNESS"=41994, "EXIF_DEVICESETTINGDESCRIPTION"=41995, "EXIF_SUBJECTDISTANCERANGE"=41996, "EXIF_IMAGEUNIQUEID"=42016, "DNGVERSION"=50706, "DNGBACKWARDVERSION"=50707, "UNIQUECAMERAMODEL"=50708, "LOCALIZEDCAMERAMODEL"=50709, "CFAPLANECOLOR"=50710, "CFALAYOUT"=50711, "LINEARIZATIONTABLE"=50712, "BLACKLEVELREPEATDIM"=50713, "BLACKLEVEL"=50714, "BLACKLEVELDELTAH"=50715, "BLACKLEVELDELTAV"=50716, "WHITELEVEL"=50717, "DEFAULTSCALE"=50718, "DEFAULTCROPORIGIN"=50719, "DEFAULTCROPSIZE"=50720, "COLORMATRIX1"=50721, "COLORMATRIX2"=50722, "CAMERACALIBRATION1"=50723, "CAMERACALIBRATION2"=50724, "REDUCTIONMATRIX1"=50725, "REDUCTIONMATRIX2"=50726, "ANALOGBALANCE"=50727, "ASSHOTNEUTRAL"=50728, "ASSHOTWHITEXY"=50729, "BASELINEEXPOSURE"=50730, "BASELINENOISE"=50731, "BASELINESHARPNESS"=50732, "BAYERGREENSPLIT"=50733, "LINEARRESPONSELIMIT"=50734, "CAMERASERIALNUMBER"=50735, "LENSINFO"=50736, "CHROMABLURRADIUS"=50737, "ANTIALIASSTRENGTH"=50738, "SHADOWSCALE"=50739, "DNGPRIVATEDATA"=50740, "MAKERNOTESAFETY"=50741, "CALIBRATIONILLUMINANT1"=50778, "CALIBRATIONILLUMINANT2"=50779, "BESTQUALITYSCALE"=50780, "RAWDATAUNIQUEID"=50781, "ORIGINALRAWFILENAME"=50827, "ORIGINALRAWFILEDATA"=50828, "ACTIVEAREA"=50829, "MASKEDAREAS"=50830, "ASSHOTICCPROFILE"=50831, "ASSHOTPREPROFILEMATRIX"=50832, "CURRENTICCPROFILE"=50833, "CURRENTPREPROFILEMATRIX"=50834, "DCSHUESHIFTVALUES"=65535, "FAXMODE"=65536, "JPEGQUALITY"=65537, "JPEGCOLORMODE"=65538, "JPEGTABLESMODE"=65539, "FAXFILLFUNC"=65540, "PIXARLOGDATAFMT"=65549, "DCSIMAGERTYPE"=65550, "DCSINTERPMODE"=65551, "DCSBALANCEARRAY"=65552, "DCSCORRECTMATRIX"=65553, "DCSGAMMA"=65554, "DCSTOESHOULDERPTS"=65555, "DCSCALIBRATIONFD"=65556, "ZIPQUALITY"=65557, "PIXARLOGQUALITY"=65558, "DCSCLIPRECTANGLE"=65559, "SGILOGDATAFMT"=65560, "SGILOGENCODE"=65561] ("tag")
      n31 = call "to.net.vi"("Variant"=w59) -> ("Array"=w60:refnum<k24>[])  [unwired: 10 in]
      n32 = invoke class="Tiff" method="SetField"(reference=w61, "tag"=w62, "value"=w60) -> (reference out=w58:refnum<k24>)  [unwired: 2 in, 4 out]
    }
    frame True {
    }
  }
  "TiffOut" <- w1
